vi "NEW数据采集传输系统.vi"() -> ()   [LabVIEW 2016, in "数据传输系统.lvlib"]
uses:
  <vilib>/Averna/Notify Icon/NotifyIcon.llb/BalloonIcon.ctl
  <vilib>/Utility/miscctls.llb/LVPointTypeDef.ctl
  <vilib>/Utility/config.llb/Read Key (String).vi
  <vilib>/Averna/Notify Icon/NotifyIcon.llb/GetSelectedItemEvent.vi
  <vilib>/Averna/Notify Icon/NotifyIcon.llb/SetVisible.vi
  <vilib>/Averna/Notify Icon/NotifyIcon.llb/SetMenuDefaultItem.vi
  <vilib>/Averna/Notify Icon/NotifyIcon.llb/SetTipText.vi
  <vilib>/Utility/config.llb/NI_LVConfig.lvlib
  data/FreeMem.dll
  <vilib>/Averna/Notify Icon/NotifyIcon.llb/NotifyIcon.lvclass
  <vilib>/ptbypt/NI_PtbyPt.lvlib
panel:
  in  "参数数值":T1={"CODMn"=TRUE, "CODCr"=TRUE, "DO"=TRUE, "铜"=TRUE, "PH"=TRUE, "氨氮"=TRUE, "比电导率"=TRUE, "水温"=TRUE, "COD"=TRUE, "浊度"=TRUE, "总氮"=TRUE, "总磷"=TRUE, "叶绿素a"=TRUE, "藻密度"=TRUE, "水位"=TRUE, "流速"=TRUE, "瞬时流量"=TRUE, "累积流量"=TRUE, "亚硝酸盐"=TRUE, "硫化物"=TRUE, "ORP"=TRUE, "铅"=TRUE, "镉"=TRUE, "锌"=TRUE, "镍"=TRUE, "锰"=TRUE, "汞"=TRUE, "气温"=TRUE, "气压"=TRUE, "风速"=TRUE, "风向"=TRUE}
  in  "配置表":bool caption="确定"
  out "配置表格":string[][](table)
  in  "updateconfiguration":T2={"主机"="27.154.58.30", "用户"="update", "密码"="std23506", "远程路径"="数据传输系统\\平台数据传输系统.exe", "下载文件名"="平台数据传输系统.exe", "软件版本"=""}
  out "标题显示":string
  in  "更新":bool
  out "错误输出":errorcluster
  in  "系统编码选择框":string(combo)="地表水质量监测"
  in  "数据发送通道":enum16{"TCP", "VISA"}(ring)
  in  "baud rate":u32=9600 caption="波特率"
  in  "VISA resource name":refnum<visa-resource-name> caption="VISA资源名称"
  in  "实时数据发送时间间隔/min":i32=1
  in  "数据组合发送":bool
  in  "日志、参数发送":bool
  in  "2011发送":bool
  in  "判断数据反馈":bool
  in  "数据发送协议":enum16{"2005-212协议", "2017-212协议"}(ring)=enum."2017-212协议"
  in  "重发时间":T3(ring)
  in  "重发日期":T4(ring)
  in  "开机启动":bool
  in  "确定更改起始时间":bool
  in  "更改起始时间":bool
  in  "数据发送起始时间":timestamp format="%<%.3X\n%Y/%m/%d>T"
  in  "每周自动重发":bool=TRUE
  in  "确定":bool
  in  "返回":bool
  in  "PW":string
  in  "MN":string
  in  "PORT":string
  in  "IP":string
  in  "站点设备":string
  in  "站点名称":string
  out "设置超时时间/min":i32=1
  out "状态信息":T5={"1st Error to Convert "=63, "步骤 "=enum."发送数据", "元素"="实时数据", "TCP服务端掉线计数"=0, "TCP掉线时间节点"="2019/05/08 15:24:17"} {"1st Error to Convert" items=["无错误", "参数错误", "内存已满", "超出区域", "文件结束", "文件已打开", "一般文件IO错误", "未找到文件", "文件权限错误", "磁盘已满", "路径副本", "打开过多文件", "未启用", "未找到资源文件", "无法添加资源", "未找到资源", "未找到图像", "图像内存错误", "画笔不存在", "配置错误类型", "配置未找到解析段", "配置解析错误", "配置内存错误", "错误外部代码格式", "错误外部代码偏移量", "外部代码不存在", "空窗口", "销毁窗口错误", "空菜单", "打印已中止", "错误打印记录", "打印驱动程序错误", "打印时窗口错误", "打印时内存错误", "打印对话框错误", "一般打印错误", "无效设备引用句柄", "设备未找到", "设备参数错误", "设备单位错误", "无法打开设备", "设备调用已中止", "一般错误", "用户已取消", "对象ID过低", "对象ID过高", "对象不在堆中", "未知的堆", "错误DefProc ID", "DefProc不在表格中", "范围外信息", "空方法", "未知信息", "不支持管理器调用", "错误地址", "连接过程中", "连接超时", "连接过程中", "不支持网络属性", "网络错误", "正在使用的地址", "系统缺少内存", "连接已中止", "连接已拒绝", "连接未建立", "连接已建立", "连接已关闭", "初始化错误（交互应用程序管理器）", "错误事件发生", "等待无约束事件发生处理程序", "事件发生队列溢出", "错误路径", "未发出信号量", "未识别类型（交互应用程序管理器）"]}
  out "数据接收超时指示灯":bool
  out "空闲时间/s":string
  out "系统时间":string
  out "实时小时数据上传":bool
  out "系统状态改变":bool
  out "软件版本":string
  out "掉线指示":bool
  out "核查数据上传":bool
  out "配置信息":T6
  in  "参数配置":bool
  out "反控数据发送":bool
  out "读取报文显示":string
  out "发送报文显示":string
  out "心跳包":bool
  out "通信状态":bool
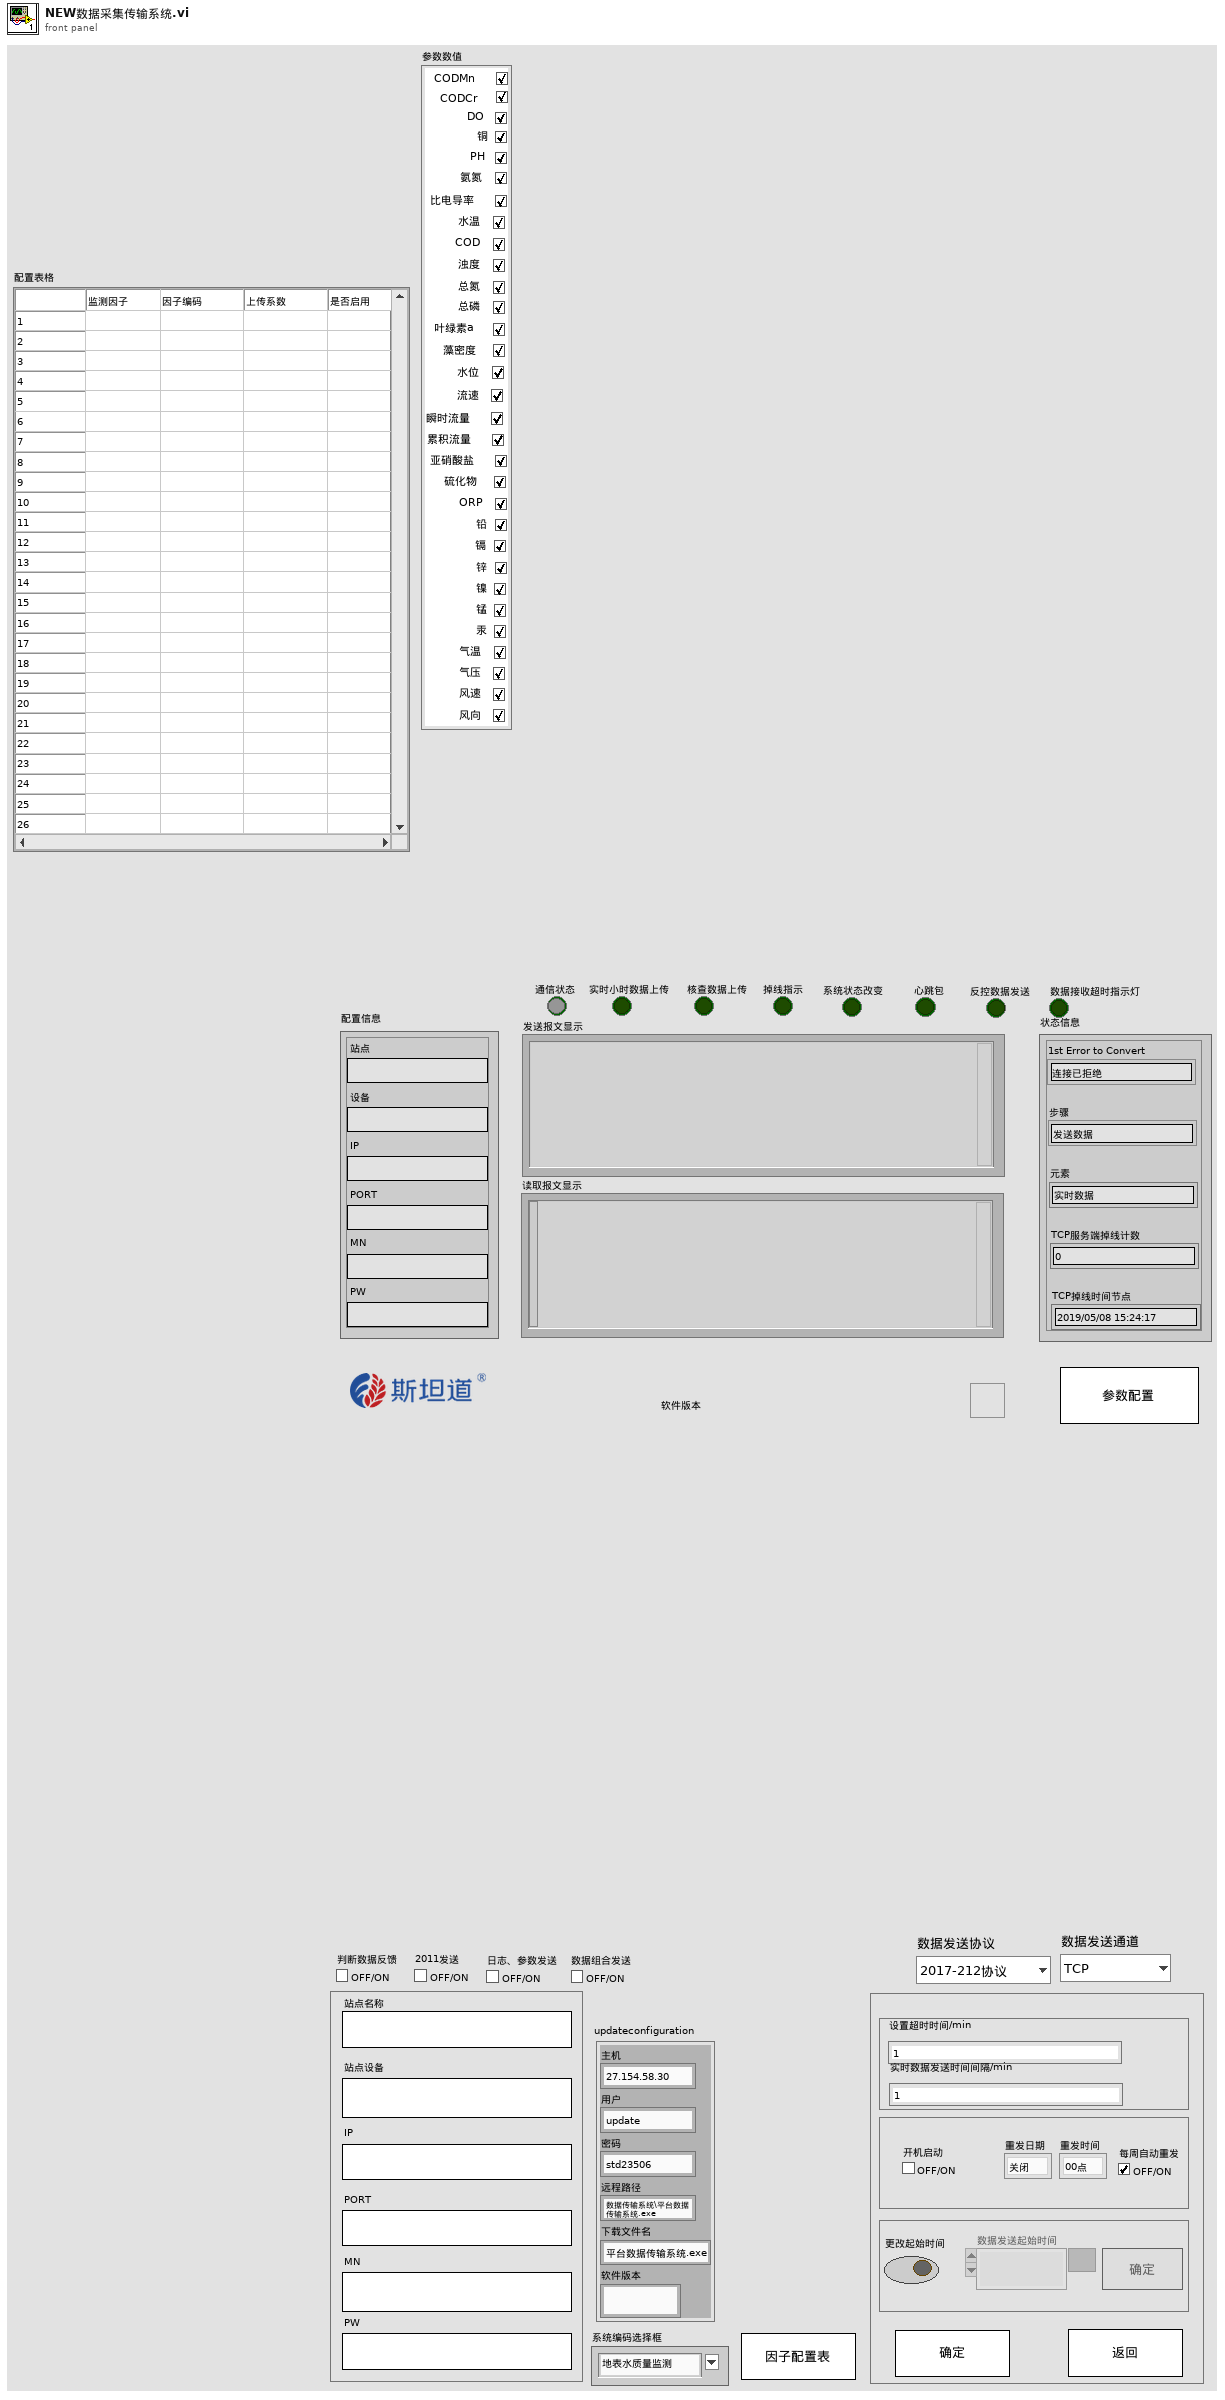
[diagram p1: front panel]
types:
  T1 = cluster{"CODMn":bool, "CODCr":bool, "DO":bool, "铜":bool, "PH":bool, "氨氮":bool, "比电导率":bool, "水温":bool, "COD":bool, "浊度":bool, "总氮":bool, "总磷":bool, "叶绿素a":bool, "藻密度":bool, "水位":bool, "流速":bool, "瞬时流量":bool, "累积流量":bool, "亚硝酸盐":bool, "硫化物":bool, "ORP":bool, "铅":bool, "镉":bool, "锌":bool, "镍":bool, "锰":bool, "汞":bool, "气温":bool, "气压":bool, "风速":bool, "风向":bool}
  T2 = cluster{"主机":string, "用户":string, "密码":string, "远程路径":string, "下载文件名":string, "软件版本":string}
  T3 = enum16{"00点", "01点", "02点", "03点", "04点", "05点", "06点", "07点", "08点", "09点", "10点", "11点", "12点", "13点", "14点", "15点", "16点", "17点", "18点", "19点", "20点", "21点", "22点", "23点"}
  T4 = enum16{"关闭", "星期日", "星期一", "星期二", "星期三", "星期四", "星期五", "星期六"}
  T5 = cluster{"1st Error to Convert ":i32, "步骤 ":enum16{"打开连接", "发送数据", "读取数据", "数据处理", "关闭连接"}, "元素":string, "TCP服务端掉线计数":i32, "TCP掉线时间节点":string}
  T6 = cluster{"站点":string, "设备":string, "IP":string, "PORT":string, "MN":string, "PW":string}
  T7 = enum32{"Invalid", "Standard", "Closed", "Hidden", "Minimized", "Maximized"}
  T8 = typedef "LVDateTimeRec.ctl" = cluster{"秒数的小数部分":dbl, "秒":i32, "分":i32, "时":i32, "日":i32, "月":i32, "年":i32, "天数（周）":i32, "天数（年）":i32, "DST":i32}
  T9 = typedef "LVPointTypeDef.ctl" = cluster{"Horizontal":i16, "Vertical":i16}
  T10 = cluster{"CODMn":string, "CODCr":string, "DO":string, "铜":string, "PH":string, "氨氮":string, "比电导率":string, "水温":string, "COD":string, "浊度":string, "总氮":string, "总磷":string, "叶绿素a":string, "藻密度":string, "水位":string, "流速":string, "瞬时流量":string, "累积流量":string, "亚硝酸盐":string, "硫化物":string, "ORP":string, "铅":string, "镉":string, "锌":string, "镍":string, "锰":string, "汞":string, "气温":string, "气压":string, "风速":string, "风向":string}
  T11 = typedef "NI_LVConfig.lvlib/Config Data RefNum.ctl" = refnum<k1>
  T12 = typedef "imagedata.ctl" = cluster{"image type":i32, "image depth":i32, "image":u8[], "mask":u8[], "colors":u32[], "Rectangle":cluster{"left":i16, "top":i16, "right":i16, "bottom":i16}}
  T13 = cluster{"[0]":string, "[1]":string, "[2]":string, "[3]":string, "[4]":string, "[5]":string, "[6]":string, "[7]":string, "[8]":string, "[9]":string, "[10]":string, "[11]":string, "[12]":string, "[13]":string, "[14]":string, "[15]":string, "[16]":string, "[17]":string, "[18]":string, "[19]":string, "[20]":string, "[21]":string, "[22]":string, "[23]":string, "[24]":string, "[25]":string, "[26]":string, "[27]":string, "[28]":string, "[29]":string, "[30]":string}
  T14 = enum8{"Enabled", "Disabled", "Disabled and Grayed Out"}
  T15 = cluster{"配置表格[0]":string, "配置表格[1]":string, "配置表格[2]":string, "配置表格[3]":string, "配置表格[4]":string, "配置表格[5]":string, "配置表格[6]":string, "配置表格[7]":string, "配置表格[8]":string, "配置表格[9]":string, "配置表格[10]":string, "配置表格[11]":string, "配置表格[12]":string, "配置表格[13]":string, "配置表格[14]":string, "配置表格[15]":string, "配置表格[16]":string, "配置表格[17]":string, "配置表格[18]":string, "配置表格[19]":string, "配置表格[20]":string, "配置表格[21]":string, "配置表格[22]":string, "配置表格[23]":string, "配置表格[24]":string, "配置表格[25]":string, "配置表格[26]":string, "配置表格[27]":string, "配置表格[28]":string, "配置表格[29]":string, "配置表格[30]":string}
  T16 = cluster{"[0]":string, "[1]":string, "[2]":string, "[3]":string, "[4]":string, "[5]":string, "[6]":string, "[7]":string}
  T17 = cluster{"[0]":string, "[1]":string, "[2]":string, "[3]":string, "[4]":string, "[5]":string, "[6]":string, "[7]":string, "[8]":string, "[9]":string, "[10]":string, "[11]":string, "[12]":string, "[13]":string, "[14]":string}
  T18 = typedef "NotifyIcon.lvlib/NotifyIcon.lvclass/BalloonIcon.ctl" = enum32{"None", "Information", "Warning", "Error"}
  T19 = enum32{"invalid app kind", "Development System", "Run Time System", "Student Edition", "Embedded LabVIEW", "Evaluation", "Custom"}
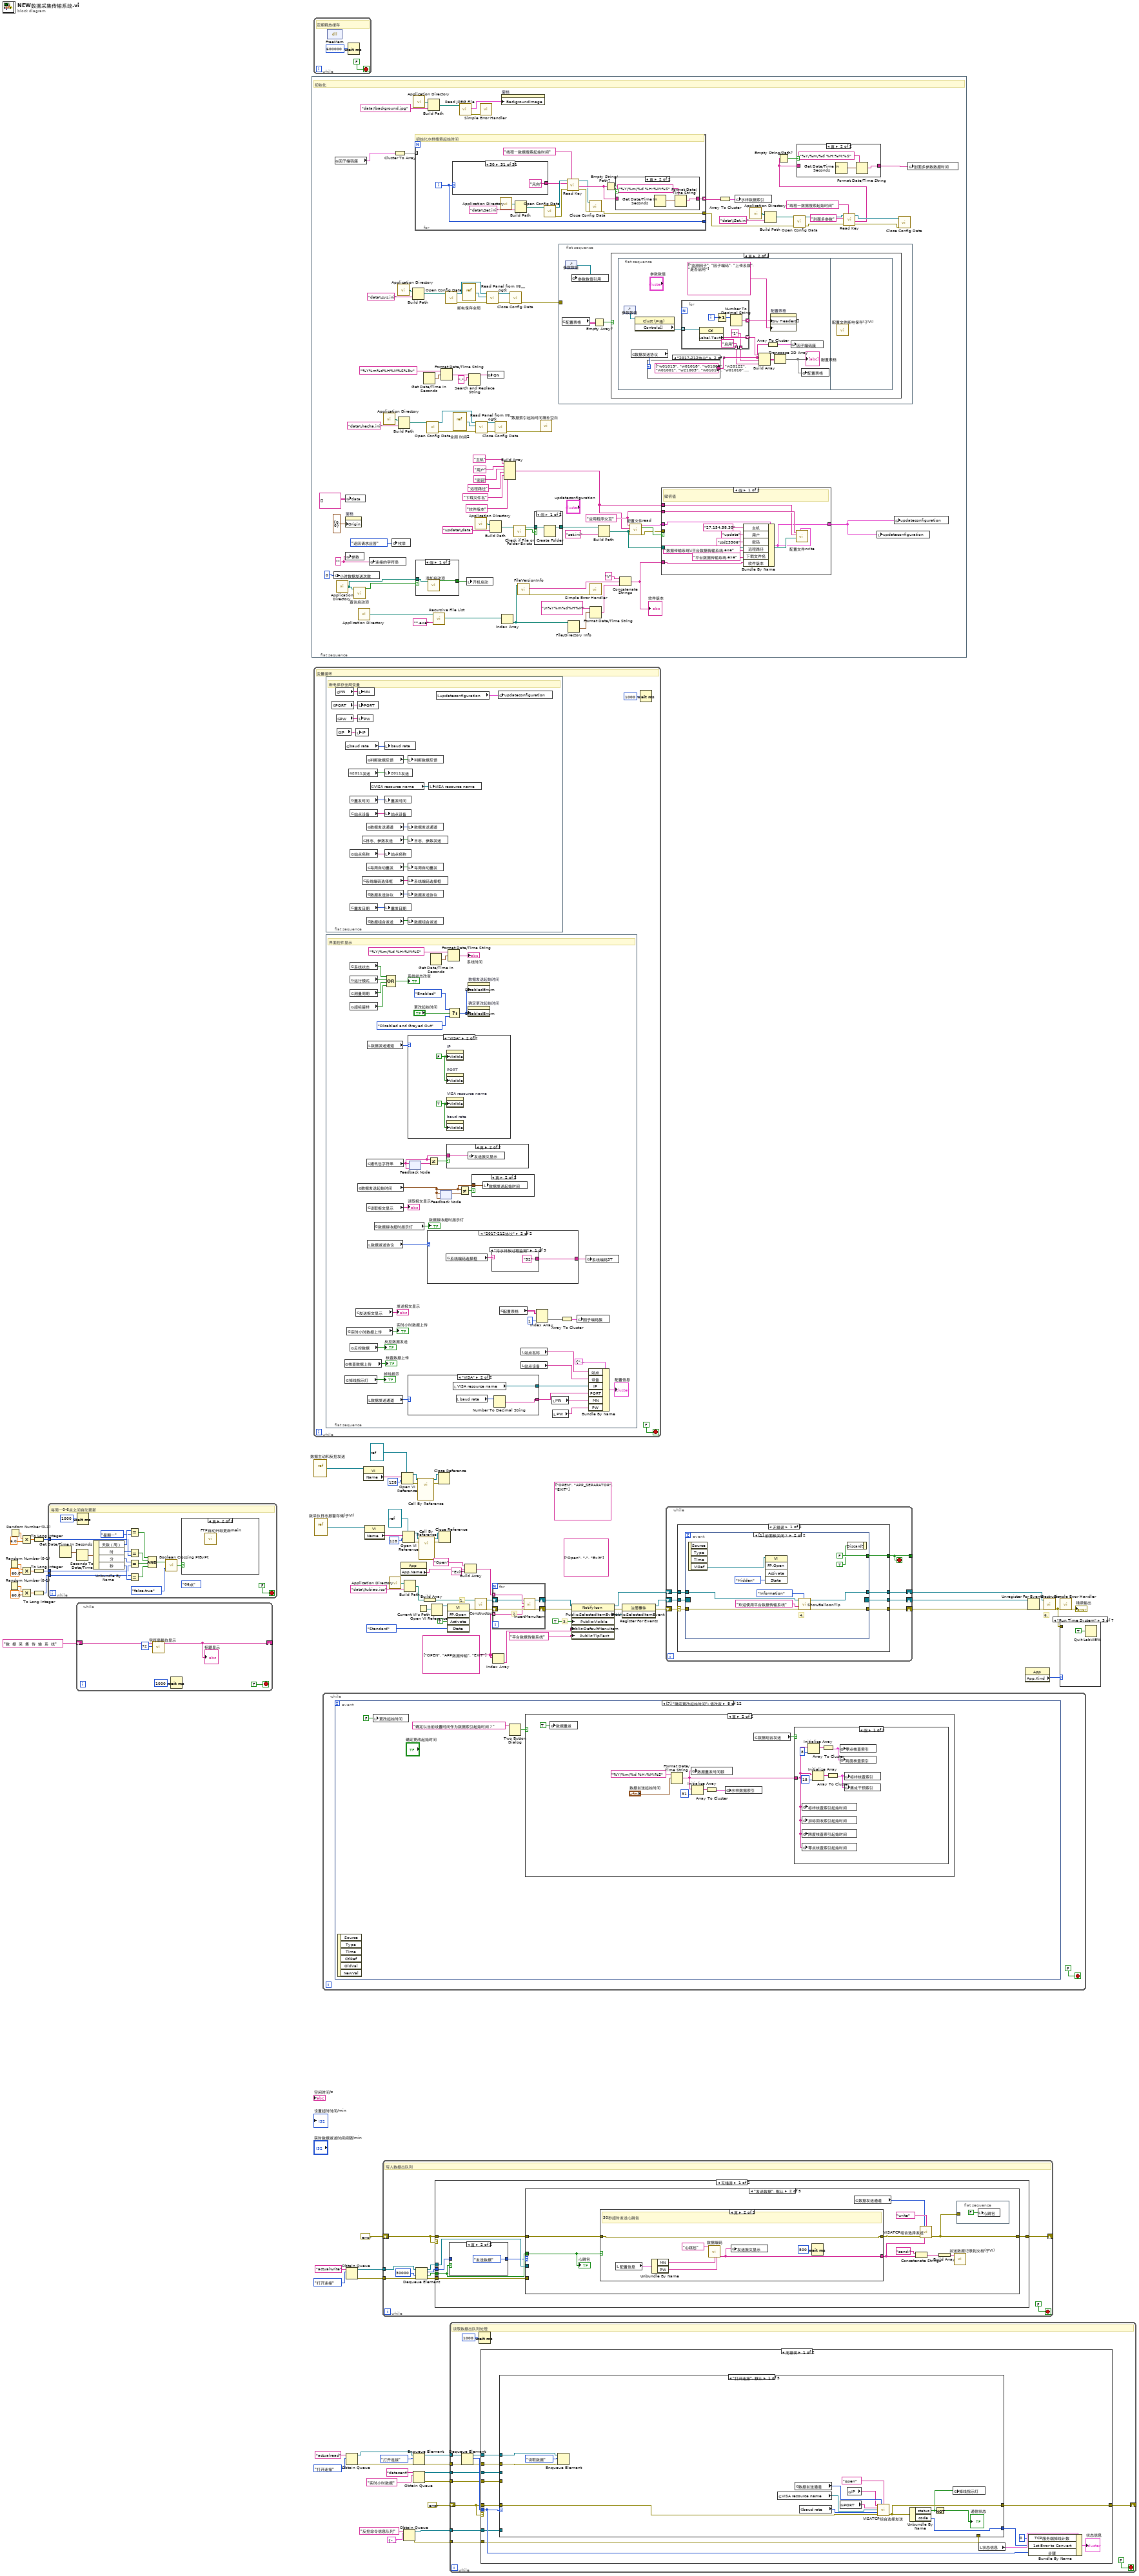
[diagram p0: block diagram]
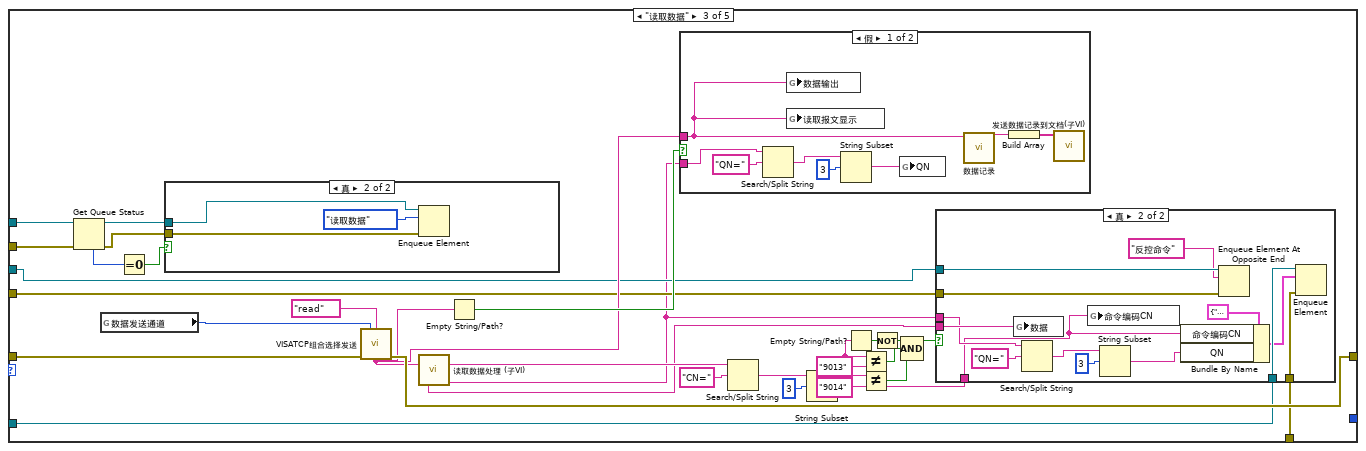
[diagram p4: hidden frame]
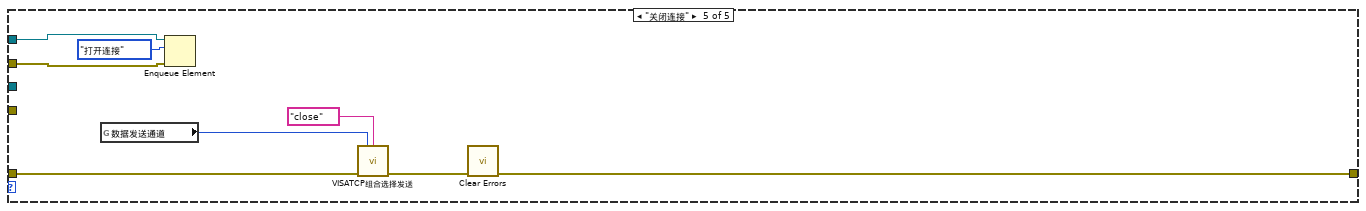
[diagram p9: hidden frame]
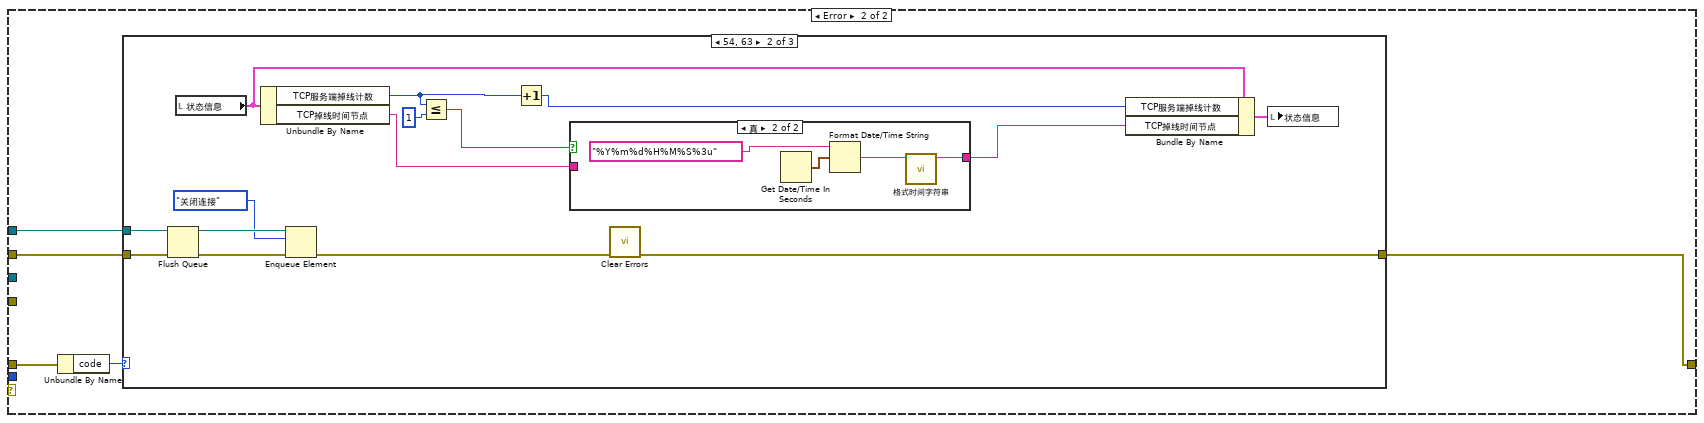
[diagram p10: hidden frame]
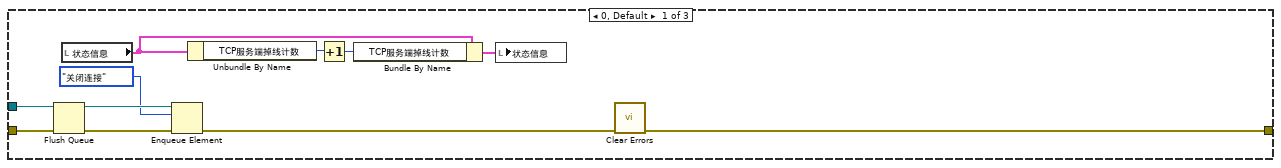
[diagram p11: hidden frame]
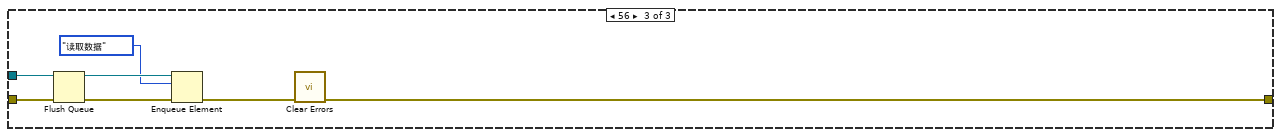
[diagram p13: hidden frame]
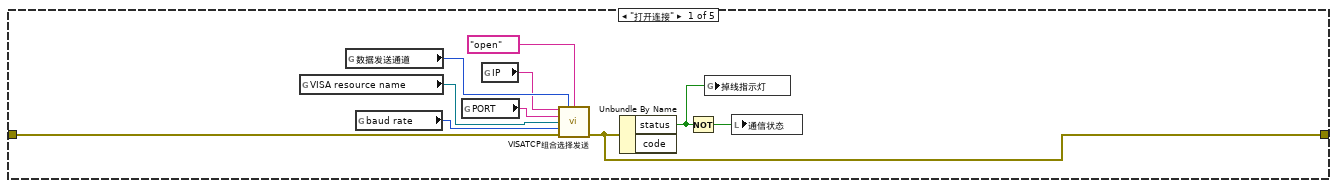
[diagram p15: hidden frame]
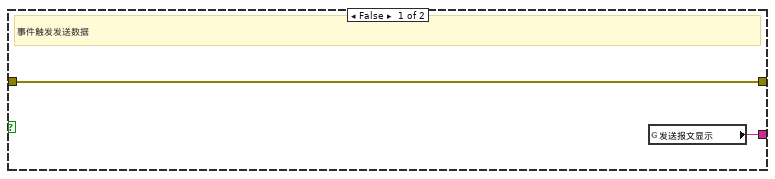
[diagram p16: hidden frame]
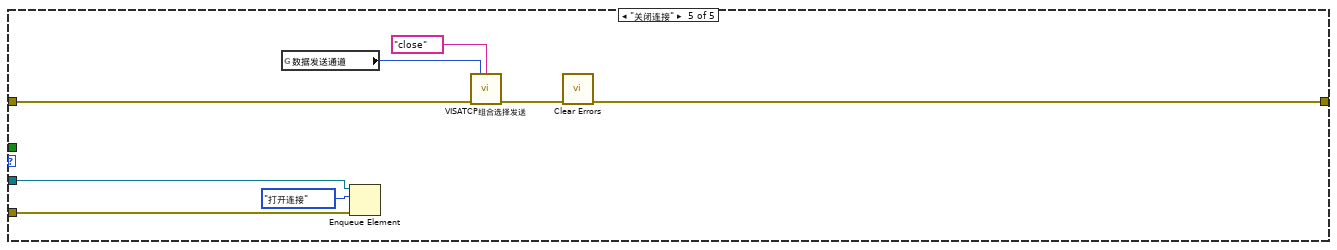
[diagram p19: hidden frame]
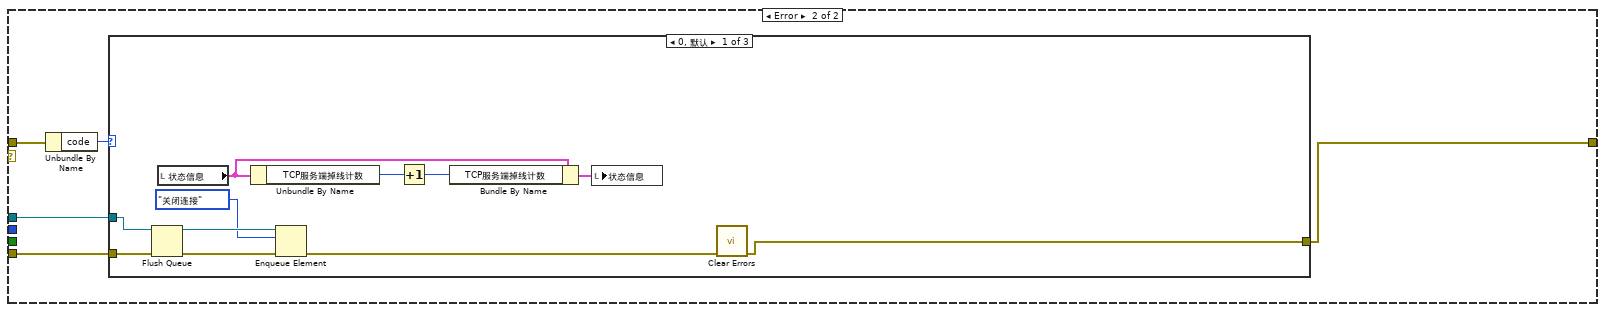
[diagram p20: hidden frame]
diagram:
  w1 = string[] ["OPEN", "APP数据传输", "EXIT"]
  (unwired) string[] ["OPEN", "APP_SEPARATOR", "EXIT"]
  (unwired) string[] ["Open", "-", "Exit"]
  # "6."
  # "3."
  # "1."
  n1 = Random Number (0-1)() -> (number: 0 to 1=w15:dbl)
  n2 = Random Number (0-1)() -> (number: 0 to 1=w14:dbl)
  n3 = Random Number (0-1)() -> (number: 0 to 1=w18:dbl)
  n4 = Multiply(x=w18, y=6.0) -> (x*y=w12:dbl)
  n5 = Multiply(x=w15, y=60.0) -> (x*y=w10:dbl)
  n6 = Multiply(x=w14, y=60.0) -> (x*y=w8:dbl)
  n7 = To Long Integer(number=w12) -> (32bit integer=w11:i32)
  n8 = To Long Integer(number=w10) -> (32bit integer=w9:i32)
  n9 = To Long Integer(number=w8) -> (32bit integer=w7:i32)
  n10 = while {
    tunnel: w11 -> [w91]
    tunnel: w9 -> [w86]
    tunnel: w7 -> [w85]
    stop <- FALSE stop-if-true
    (unwired) T3."06点" ("重发时间")
    # "每周一0-6点之间自动更新"
    n11 = Get Date/Time In Seconds() -> (seconds since 1Jan1904=w100:timestamp)
    n12 = Seconds To Date/Time(time stamp (now)=w100) -> (date time rec=w96:T8)  [unwired: 1 in]
    n13 = Wait (ms)(milliseconds to wait=u32 1000 ("等待时间（毫秒）")) -> ()  [unwired: 1 out]
    n14 = Unbundle By Name(w96) -> ("天数（周）"=w99:i32, "时"=w93:i32, "分"=w90:i32, "秒"=w88:i32)
    n15 = Equal?(x=w99, y=T4."星期一" ("重发日期")) -> (x = y?=w98:bool)
    n16 = Equal?(x=w93, y=w91) -> (x = y?=w97:bool)
    n17 = Equal?(x=w90, y=w86) -> (x = y?=w89:bool)
    n18 = Equal?(x=w85, y=w88) -> (x = y?=w87:bool)
    n19 = Compound Arithmetic op=AND ("复合运算")(w98, w97, w89, w87) -> (w95:bool)
    n20 = call <vilib>:"Boolean Crossing PtByPt.vi"("direction"=enum16{"either", "false-true", "true-false"}."false-true", "input"=w95) -> ("crossing"=w84:bool)  [unwired: 1 in]
    n21 = case shown="真" w84 {
      frame False {
      }
      frame True {
        n22 = call "FTP自动升级更新main.vi"() -> ()  [unwired: 12 in]
      }
    }
  }
  n23 = while {
    shift-right: [w104] -> _
    shift-left: "数  据  采  集  传  输  系  统" ("标题显示") -> [w105]
    stop <- FALSE stop-if-true
    n24 = call "字符串移位显示.vi"("字符框大小"=72, "字符串输入"=w105) -> ("移位后字符串"=w104:string)  [unwired: 8 in, 1 out]
    "标题显示" <- w104
    n25 = Wait (ms)(milliseconds to wait=u32 1000 ("等待时间（毫秒）")) -> ()  [unwired: 1 out]
  }
  n26 = flat-sequence {
    frame #0 {
      w142 = "应用程序交互" ("section")
      w189 = "" ("参数")
      # "初始化"
      n27 = global write "全局 小时数据发送次数.vi" "小时数据发送次数"(0 ("数值")) -> ()
      n28 = global read "断电保存全局.vi" "因子编码簇"() -> (w108:T10)
      n29 = call <vilib>:"Application Directory.vi"() -> ("Application Directory"=w111:path)
      n30 = global write "全局 实时数据参数.vi" "data"(string[][] [] ("data")) -> ()
      n31 = property on="窗格" class="Pane"("Origin"=T9 {"Horizontal"=0, "Vertical"=0} ("原点")) -> ()  [unwired: 2 in, 2 out]
      n32 = global write "全局 实时数据参数.vi" "参数"(w189) -> ()
      n33 = call "查询启动项.vi"("启动文件路径"=w111) -> ("包含启动项"=w112:bool)  [unwired: 9 in, 1 out]
      n34 = call <vilib>:"Application Directory.vi"() -> ("Application Directory"=w169:path)
      n35 = global write "全局 实时数据参数.vi" "连接的字符串"(w189) -> ()
      n36 = call <vilib>:"Application Directory.vi"() -> ("Application Directory"=w155:path)
      n37 = global write "全局1.vi" "枚举"(enum16{"返回请求应答", "上传数据", "返回执行结果"}."返回请求应答" ("枚举")) -> ()
      n38 = Cluster To Array(cluster=w108) -> (array=w148:string[])
      n39 = call <vilib>:"Application Directory.vi"() -> ("Application Directory"=w163:path)
      n40 = Build Path(base path=w155, name or relative path="data\\hecha.ini" ("名称或相对路径")) -> (appended path=w157:path)
      n41 = Build Path(base path=w163, name or relative path="data\\sys.ini" ("名称或相对路径")) -> (appended path=w161:path)
      n42 = call <vilib>:"Application Directory.vi"() -> ("Application Directory"=w180:path)
      n43 = for {
        tunnel: w148 -> [_] mode=indexing
        tunnel: [w248] -> _
        tunnel: [w245] -> w147 mode=indexing
        tunnel: [w244] -> w122
        i -> [w248]
        # "初始化水样搜索起始时间"
        n44 = case shown="30" w248 {
          tunnel: ["CODMn" "CODCr" "DO" "铜" "PH" "氨氮" "比电导率" "水温" "COD" "浊度" "总氮" "总磷" "叶绿素a" "藻密度" "水位" "流速" "瞬时流量" "累积流量" "亚硝氮" "硫化物" "ORP" "铅" "镉" "锌" "镍" "锰" "汞" "气温" "气压" "风速" "风向"] -> w251
          frame 0, Default {
          }
          frame 1 {
          }
          frame 2 {
          }
          frame 3 {
          }
          frame 4 {
          }
          frame 5 {
          }
          frame 6 {
          }
          frame 7 {
          }
          frame 8 {
          }
          frame 9 {
          }
          frame 10 {
          }
          frame 11 {
          }
          frame 12 {
          }
          frame 13 {
          }
          frame 14 {
          }
          frame 15 {
          }
          frame 16 {
          }
          frame 17 {
          }
          frame 18 {
          }
          frame 19 {
          }
          frame 20 {
          }
          frame 21 {
          }
          frame 22 {
          }
          frame 23 {
          }
          frame 24 {
          }
          frame 25 {
          }
          frame 26 {
          }
          frame 27 {
          }
          frame 28 {
          }
          frame 29 {
          }
          frame 30 {
          }
        }
        n45 = call <vilib>:"Application Directory.vi"() -> ("Application Directory"=w257:path)
        n46 = Build Path(base path=w257, name or relative path="data\\Set.ini" ("名称或相对路径")) -> (appended path=w255:path)
        n47 = call <vilib>:"Open Config Data.vi"("configuration file path"=w255) -> ("error out"=w253:errorcluster, "refnum"=w254:T11)  [unwired: 8 in, 1 out]
        n48 = call-poly <vilib>:"Read Key.vi"("section"="线程一数据搜索起始时间", "error in (no error)"=w253, "key"=w251, "refnum"=w254) -> ("error out"=w246:errorcluster, "value"=w249:string, "refnum out"=w247:T11)  [unwired: 4 in, 1 out]
        n49 = call <vilib>:"Close Config Data.vi"("error in (no error)"=w246, "refnum"=w247) -> ("error out"=w244:errorcluster)  [unwired: 8 in, 1 out]
        n50 = Empty String/Path?(string/path=w249) -> (empty?=w250:bool)
        n51 = case shown="真" w250 {
          tunnel: [w258 w259] -> w245
          tunnel: w249 -> [w258 _]
          frame False {
          }
          frame True {
            n52 = Get Date/Time In Seconds() -> (seconds since 1Jan1904=w261:timestamp)
            n53 = Format Date/Time String(time format string (%c)="%Y/%m/%d %H:%M:%S" ("时间格式字符串(%c)"), seconds (now)=w261) -> (date/time string=w259:string)  [unwired: 1 in]
          }
        }
      }
      n54 = case shown="假" w112 {
        selector: w112 -> [_ w218]
        tunnel: w111 -> [w217 _]
        tunnel: [w216 w218] -> w110
        frame False {
          n55 = call "添加启动项.vi"("启动文件路径"=w217) -> ("添加成功标记"=w216:bool)  [unwired: 9 in, 1 out]
        }
        frame True {
        }
      }
      n56 = Get Date/Time In Seconds() -> (seconds since 1Jan1904=w185:timestamp)
      n57 = call <vilib>:"Open Config Data.vi"("configuration file path"=w157) -> ("error out"=w151:errorcluster, "refnum"=w152:T11)  [unwired: 8 in, 1 out]
      n58 = Build Path(base path=w180, name or relative path="data\\background.jpg" ("名称或相对路径")) -> (appended path=w179:path)
      n59 = call <vilib>:"Recursive File List.vi"("pattern"="*.exe", "Folder Path"=w169) -> ("All Files in Dir"=w175:path[])  [unwired: 5 in, 4 out]
      n60 = Format Date/Time String(time format string (%c)="%Y%m%d%H%M%S%3u" ("时间格式字符串(%c)"), seconds (now)=w185) -> (date/time string=w184:string)  [unwired: 1 in]
      n61 = call <vilib>:"Open Config Data.vi"("configuration file path"=w161) -> ("error out"=w167:errorcluster, "refnum"=w166:T11)  [unwired: 8 in, 1 out]
      n62 = vi-ref "全局 时间2.vi"() -> (w153:refnum<vi>)
      n63 = call <vilib>:"Read JPEG File.vi"("path to JPEG file"=w179) -> ("error out"=w177:errorcluster, "image data"=w178:T12)  [unwired: 8 in, 1 out]
      n64 = vi-ref "断电保存全局.vi"() -> (w165:refnum<vi>)
      n65 = local write "开机启动"(w110) -> ()
      n66 = Search and Replace String(input string=w184, search string="." ("搜索字符串")) -> (result string=w182:string)  [unwired: 6 in, 3 out]
      n67 = call <vilib>:"Application Directory.vi"() -> ("Application Directory"=w128:path)
      n68 = call <userlib>:"Read Panel from INI__ogtk.vi"("error in (no error)"=w151, "VI ref"=w153, "refnum"=w152) -> ("error out"=w150:errorcluster, "refnum out"=w154:T11)  [unwired: 7 in]
      n69 = call <vilib>:"Simple Error Handler.vi"("error in (no error)"=w177) -> ()  [unwired: 4 in, 5 out]
      n70 = call <userlib>:"Read Panel from INI__ogtk.vi"("error in (no error)"=w167, "VI ref"=w165, "refnum"=w166) -> ("error out"=w160:errorcluster, "refnum out"=w164:T11)  [unwired: 7 in]
      n71 = global write "全局1.vi" "QN"(w182) -> ()
      n72 = Build Path(base path=w128, name or relative path="update\\data" ("名称或相对路径")) -> (appended path=w129:path)
      n73 = call <vilib>:"Close Config Data.vi"("error in (no error)"=w150, "refnum"=w154) -> ("error out"=w149:errorcluster)  [unwired: 8 in, 1 out]
      n74 = property on="窗格" class="Pane"("BackgroundImage"=w178) -> ()  [unwired: 2 in, 2 out]
      n75 = Index Array(array=w175) -> (element=w174:path)  [unwired: 1 in]
      n76 = Build Array("主机" ("section"), "用户" ("section"), "密码" ("key"), "远程路径" ("key"), "下载文件名" ("key"), "软件版本" ("key")) -> (w132:string[])
      n77 = call <vilib>:"Close Config Data.vi"("error in (no error)"=w160, "refnum"=w164) -> ("error out"=w109:errorcluster)  [unwired: 8 in, 1 out]
      n78 = call <vilib>:"Check if File or Folder Exists.vi"("path"=w129) -> ("file or folder exists?"=w130:bool, "dup path"=w131:path)  [unwired: 8 in, 1 out]
      n79 = call <vilib>:"FileVersionInfo.vi"("Application Path in"=w174) -> ("error out"=w168:errorcluster, "File Version Info"=w158:string)  [unwired: 7 in, 2 out]
      n80 = case shown="假" w130 {
        tunnel: w131 -> [w224 w225]
        tunnel: [w223 w225] -> w126
        frame False {
          n81 = Create Folder(path (use dialog)=w224) -> (created path=w223:path)  [unwired: 2 in, 2 out]
        }
        frame True {
        }
      }
      n82 = call "数据索引起始时间填补空白.vi"("error in (no error)"=w149) -> ()  [unwired: 10 in, 1 out]
      n83 = flat-sequence {
        tunnel: w109 -> [_]
        frame #0 {
          n84 = global read "断电保存全局.vi" "配置表格"() -> (w194:string[][])
          n85 = control-ref of="参数数值"() -> (w192:refnum<vi>)
          n86 = global write "断电保存全局.vi" "参数数值引用"(w192) -> ()
          n87 = Empty Array?(array=w194) -> (empty?=w193:bool)
          n88 = case shown="真" w193 {
            frame False {
            }
            frame True {
              n89 = flat-sequence {
                frame #0 {
                  n90 = control-ref of="参数数值"() -> (w195:refnum<vi>)
                  n91 = global read "断电保存全局.vi" "数据发送协议"() -> (w200:enum16{"2005-212协议", "2017-212协议"})
                  n92 = property on="属性节点" class="Clust (严格)"(reference=w195) -> ("Controls[]"=w202:refnum<vi>[])  [unwired: 1 in, 2 out]
                  n93 = case shown="\"2017-212协议\"" w200 {
                    tunnel: [string[] ["w01019", "011", "w01009", "w20122", "001", "060", "w01014", "w01010", "w01018", "w01003", "065", "101", "w01016", "w19011", "e01201", "e01202", "B01", "e01204", "w21006", "w21019", "w01100", "w20120", "w20115", "w20123", "w20121", "w20124", "w20111"] string[] ["w01019", "w01018", "w01009", "w20122", "w01001", "w21003", "w01014", "w01010", "w01018", "w01003", "w21001", "w21011", "w01016", "w19011", "e01201", "e01202", "e01203", "e01204", "w21006", "w21019", "w01100", "w20120", "w20115", "w20123", "w20121", "w20124", "w20111"]] -> w198
                    frame "2005-212协议", Default {
                    }
                    frame "2017-212协议" {
                    }
                  }
                  n94 = for {
                    tunnel: w202 -> [w215] mode=indexing
                    tunnel: [w214] -> w204 mode=indexing
                    tunnel: [w212] -> w203 mode=indexing
                    tunnel: ["1"] -> w197 mode=indexing
                    tunnel: ["启用"] -> w196 mode=indexing
                    i -> [w213]
                    n95 = property class="Ctl"(reference=w215) -> ("Label.Text"=w214:string)  [unwired: 1 in, 2 out]
                    n96 = Increment(x=w213) -> (x+1=w211:i32)
                    n97 = Number To Decimal String(number=w211) -> (decimal integer string=w212:string)  [unwired: 1 in]
                  }
                  n98 = Build Array(w204, w198, w197, w196) -> (w206:string[][])
                  n99 = Array To Cluster(array=w198) -> (cluster=w199:T13)
                  n100 = property on="配置表格" class="Tbl (严格)"("Row Headers[]"=w203, "Column Headers[]"=string[] ["监测因子", "因子编码", "上传系数", "是否启用"]) -> ()  [unwired: 2 in, 2 out]
                  n101 = Transpose 2D Array(2D array=w206) -> (transposed array=w201:string[][])
                  "配置表格" <- w201
                  n102 = global write "断电保存全局.vi" "因子编码簇"(w199) -> ()
                  n103 = global write "断电保存全局.vi" "配置表格"(w201) -> ()
                }
                frame #1 {
                  n104 = call "配置文件断电保存(子VI).vi"() -> ()  [unwired: 12 in]
                }
              }
            }
          }
        }
      }
      n105 = File/Directory Info(path=w174) -> (last mod=w173:timestamp)  [unwired: 1 in, 6 out]
      n106 = call <vilib>:"Simple Error Handler.vi"("error in (no error)"=w168) -> ()  [unwired: 4 in, 5 out]
      n107 = Format Date/Time String(time format string (%c)="\n%Y%m%d%H%M" ("时间格式字符串(%c)"), seconds (now)=w173) -> (date/time string=w170:string)  [unwired: 1 in]
      n108 = Build Path(base path=w126, name or relative path="set.ini" ("名称或相对路径")) -> (appended path=w141:path)
      n109 = Concatenate Strings("V" ("字符串"), w158, w170) -> (w143:string)
      "软件版本" <- w143
      n110 = call "配置文件read.vi"("configuration file path"=w141, "键数组"=w132, "段"=w142) -> ("error out"=w140:errorcluster, "section exists?"=w145:bool, "updateconfiguration"=w144:T2)  [unwired: 6 in]
      n111 = case shown="假" w145 {
        tunnel: w144 -> [w232 w238]
        tunnel: [w231 w237] -> w139
        tunnel: w143 -> [w226 w243]
        tunnel: w142 -> [w235 w242]
        tunnel: w132 -> [w234 w241]
        tunnel: w141 -> [w233 w240]
        tunnel: w140 -> [_ w239]
        frame False {
          # "赋初值"
          n112 = Bundle By Name(cluster=w232, "主机"="27.154.58.30" ("key"), "用户"="update", "密码"="std23506", "远程路径"="数据传输系统\\平台数据传输系统.exe", "下载文件名"="平台数据传输系统.exe", "软件版本"=w226) -> (w231:T2)
          n113 = call "配置文件write.vi"("updateconfiguration"=w231, "configuration file path"=w233, "键数组"=w234, "段"=w235) -> ()  [unwired: 7 in, 1 out]
        }
        frame True {
          # "本地"
          n114 = Bundle By Name(cluster=w238, "软件版本"=w243) -> (w237:T2)
          n115 = call "配置文件write.vi"("updateconfiguration"=w237, "error in (no error)"=w239, "configuration file path"=w240, "键数组"=w241, "段"=w242) -> ()  [unwired: 6 in, 1 out]
        }
      }
      n116 = Array To Cluster(array=w147) -> (cluster=w146:T13)
      n117 = global write "全局 水样时间.vi" "水样数据索引"(w146) -> ()
      n118 = call <vilib>:"Application Directory.vi"() -> ("Application Directory"=w125:path)
      n119 = Build Path(base path=w125, name or relative path="data\\Set.ini" ("名称或相对路径")) -> (appended path=w123:path)
      n120 = call <vilib>:"Open Config Data.vi"("error in (no error)"=w122, "configuration file path"=w123) -> ("error out"=w119:errorcluster, "refnum"=w120:T11)  [unwired: 7 in, 1 out]
      n121 = call-poly <vilib>:"Read Key.vi"("section"="线程一数据搜索起始时间", "error in (no error)"=w119, "key"="剖面多参数", "refnum"=w120) -> ("error out"=w116:errorcluster, "value"=w114:string, "refnum out"=w117:T11)  [unwired: 4 in, 1 out]
      n122 = Empty String/Path?(string/path=w114) -> (empty?=w113:bool)
      n123 = case shown="真" w113 {
        tunnel: [w219 w220] -> w115
        tunnel: w114 -> [w219 _]
        frame False {
        }
        frame True {
          n124 = Get Date/Time In Seconds() -> (seconds since 1Jan1904=w222:timestamp)
          n125 = Format Date/Time String(time format string (%c)="%Y/%m/%d %H:%M:%S" ("时间格式字符串(%c)"), seconds (now)=w222) -> (date/time string=w220:string)  [unwired: 1 in]
        }
      }
      n126 = local write "updateconfiguration"(w139) -> ()
      n127 = global write "update全局.vi" "updateconfiguration"(w139) -> ()
      n128 = call <vilib>:"Close Config Data.vi"("error in (no error)"=w116, "refnum"=w117) -> ()  [unwired: 8 in, 2 out]
      n129 = global write "全局 水样时间.vi" "剖面多参数数据时间"(w115) -> ()
    }
  }
  n130 = while {
    stop <- FALSE stop-if-true
    # "定期释放缓存"
    n131 = dll-call lib="PTH2aabs F\tgitkrakenCC6平台数采程序 - V2.0.1（正式修改迭代版）dataFreeMem.dll" fn="FreeMem"() -> ()  [unwired: 4 in, 2 out]
    n132 = Wait (ms)(milliseconds to wait=u32 600000 ("等待时间（毫秒）")) -> ()  [unwired: 1 out]
  }
  n133 = while {
    stop <- FALSE stop-if-true
    # "变量循环"
    n134 = flat-sequence {
      frame #0 {
        # "断电保存全局变量"
        n135 = global read "断电保存全局.vi" "PORT"() -> (w370:string)
        n136 = global read "断电保存全局.vi" "MN"() -> (w369:string)
        n137 = global read "断电保存全局.vi" "PW"() -> (w368:string)
        n138 = global read "断电保存全局.vi" "IP"() -> (w371:string)
        n139 = global read "断电保存全局.vi" "baud rate"() -> (w366:u32)
        n140 = global read "断电保存全局.vi" "2011发送"() -> (w362:bool)
        n141 = global read "断电保存全局.vi" "重发时间"() -> (w356:T3)
        n142 = global read "断电保存全局.vi" "站点设备"() -> (w372:string)
        n143 = global read "断电保存全局.vi" "站点名称"() -> (w373:string)
        n144 = global read "断电保存全局.vi" "重发日期"() -> (w364:T4)
        n145 = local write "IP"(w371) -> ()
        n146 = local write "MN"(w369) -> ()
        n147 = local write "PORT"(w370) -> ()
        n148 = local write "PW"(w368) -> ()
        n149 = global read "断电保存全局.vi" "日志、参数发送"() -> (w361:bool)
        n150 = global read "断电保存全局.vi" "系统编码选择框"() -> (w357:string)
        n151 = global read "断电保存全局.vi" "判断数据反馈"() -> (w363:bool)
        n152 = global read "断电保存全局.vi" "数据发送通道"() -> (w358:enum16{"TCP", "VISA"})
        n153 = global read "断电保存全局.vi" "每周自动重发"() -> (w365:bool)
        n154 = global read "断电保存全局.vi" "数据发送协议"() -> (w359:enum16{"2005-212协议", "2017-212协议"})
        n155 = global read "断电保存全局.vi" "数据组合发送"() -> (w360:bool)
        n156 = global read "断电保存全局.vi" "VISA resource name"() -> (w367:refnum<visa-resource-name>)
        n157 = local write "baud rate"(w366) -> ()
        n158 = local write "2011发送"(w362) -> ()
        n159 = local write "重发时间"(w356) -> ()
        n160 = local write "站点设备"(w372) -> ()
        n161 = local write "站点名称"(w373) -> ()
        n162 = local write "重发日期"(w364) -> ()
        n163 = local write "判断数据反馈"(w363) -> ()
        n164 = local write "数据发送通道"(w358) -> ()
        n165 = local write "日志、参数发送"(w361) -> ()
        n166 = local write "每周自动重发"(w365) -> ()
        n167 = local write "系统编码选择框"(w357) -> ()
        n168 = local write "数据发送协议"(w359) -> ()
        n169 = local write "数据组合发送"(w360) -> ()
        n170 = local write "VISA resource name"(w367) -> ()
        n171 = local read "updateconfiguration"() -> (w355:T2)
        n172 = global write "update全局.vi" "updateconfiguration"(w355) -> ()
      }
    }
    n173 = flat-sequence {
      frame #0 {
        # "界面控件显示"
        n174 = global read "全局1.vi" "核查数据上传"() -> (→"核查数据上传":bool)
        n175 = global read "全局 数据发送重叠.vi" "掉线指示灯"() -> (→"掉线指示":bool)
        n176 = global read "全局1.vi" "实时小时数据上传"() -> (→"实时小时数据上传":bool)
        n177 = global read "全局1.vi" "系统状态"() -> (w304:bool)
        n178 = global read "全局1.vi" "运行模式"() -> (w305:bool)
        n179 = global read "全局1.vi" "测量周期"() -> (w306:bool)
        n180 = global read "全局1.vi" "超标留样"() -> (w307:bool)
        n181 = global read "全局1.vi" "反控数据"() -> (→"反控数据发送":bool)
        n182 = global read "全局1.vi" "发送报文显示"() -> (→"发送报文显示":string)
        n183 = global read "全局1.vi" "数据发送起始时间"() -> (w301:timestamp)
        n184 = global read "全局1.vi" "通讯包字符串"() -> (w318:string)
        n185 = global read "全局1.vi" "读取报文显示"() -> (→"读取报文显示":string)
        n186 = local read "数据发送通道"() -> (w312:enum16{"TCP", "VISA"})
        n187 = local read "数据发送协议"() -> (w326:enum16{"2005-212协议", "2017-212协议"})
        n188 = local read "数据发送通道"() -> (w337:enum16{"TCP", "VISA"})
        n189 = global read "全局 数据发送重叠.vi" "数据接收超时指示灯"() -> (→"数据接收超时指示灯":bool)
        n190 = Compound Arithmetic op=OR ("复合运算")(w304, w305, w306, w307) -> (→"系统状态改变":bool)
        n191 = case shown="\"VISA\"" w312 {
          frame "TCP", Default {
            w339 = TRUE ("可见")
            w340 = FALSE ("可见")
            n192 = property on="IP" class="Str"("Visible"=w339) -> ()  [unwired: 2 in, 2 out]
            n193 = property on="PORT" class="Str"("Visible"=w339) -> ()  [unwired: 2 in, 2 out]
            n194 = property on="VISA resource name" class="VISAName"("Visible"=w340) -> ()  [unwired: 2 in, 2 out]
            n195 = property on="baud rate" class="DigNum (严格)"("Visible"=w340) -> ()  [unwired: 2 in, 2 out]
          }
          frame "VISA" {
            w341 = FALSE ("可见")
            w342 = TRUE ("可见")
            n196 = property on="IP" class="Str"("Visible"=w341) -> ()  [unwired: 2 in, 2 out]
            n197 = property on="PORT" class="Str"("Visible"=w341) -> ()  [unwired: 2 in, 2 out]
            n198 = property on="VISA resource name" class="VISAName"("Visible"=w342) -> ()  [unwired: 2 in, 2 out]
            n199 = property on="baud rate" class="DigNum (严格)"("Visible"=w342) -> ()  [unwired: 2 in, 2 out]
          }
        }
        n200 = case shown="\"VISA\"" w337 {
          tunnel: [w351 w354] -> w334
          tunnel: [w350 w352] -> w331
          frame "TCP", Default {
            n201 = local read "PORT"() -> (w350:string)
            n202 = local read "IP"() -> (w351:string)
          }
          frame "VISA" {
            n203 = local read "VISA resource name"() -> (w354:refnum<visa-resource-name>)
            n204 = local read "baud rate"() -> (w353:u32)
            n205 = Number To Decimal String(number=w353) -> (decimal integer string=w352:string)  [unwired: 1 in]
          }
        }
        n206 = feedback #1(w318) -> (w319:string)
        n207 = feedback-in #1(w318) -> ()
        n208 = case shown="\"2017-212协议\"" w326 {
          tunnel: ["32" ("设备编码MN") w345] -> w325
          frame "2005-212协议", Default {
          }
          frame "2017-212协议" {
            n209 = global read "断电保存全局.vi" "系统编码选择框"() -> (w346:string)
            n210 = case shown="\"污水排放过程监测\"" w346 {
              tunnel: ["52" ("设备编码MN") "32" ("设备编码MN") "21" ("设备编码MN")] -> w345
              frame "污水排放过程监测" {
              }
              frame "地表水体污染源" {
              }
              frame "地表水质量监测", Default {
              }
            }
          }
        }
        n211 = Not Equal?(x=w318, y=w319) -> (x != y?=w317:bool)
        n212 = Get Date/Time In Seconds() -> (seconds since 1Jan1904=w327:timestamp)
        n213 = feedback #2(w301) -> (w303:timestamp)
        n214 = feedback-in #2(w301) -> ()
        n215 = case shown="真" w317 {
          tunnel: w318 -> [_ w343]
          frame False {
          }
          frame True {
            n216 = global write "全局1.vi" "发送报文显示"(w343) -> ()
          }
        }
        n217 = Format Date/Time String(time format string (%c)="%Y/%m/%d %H:%M:%S" ("时间格式字符串(%c)"), seconds (now)=w327) -> (date/time string=→"系统时间":string)  [unwired: 1 in]
        n218 = Select(t=T14."Enabled" ("禁用"), s="更改起始时间", f=T14."Disabled and Grayed Out" ("禁用")) -> (s? t:f=w313:T14)
        n219 = Not Equal?(x=w301, y=w303) -> (x != y?=w302:bool)
        n220 = property on="数据发送起始时间" class="AbsTime (严格)"("DisabledEnum"=w313) -> ()  [unwired: 2 in, 2 out]
        n221 = property on="确定更改起始时间" class="Bool"("DisabledEnum"=w313) -> ()  [unwired: 2 in, 2 out]
        n222 = case shown="真" w302 {
          tunnel: w301 -> [_ w338]
          frame False {
          }
          frame True {
            n223 = local write "数据发送起始时间"(w338) -> ()
          }
        }
        n224 = global read "断电保存全局.vi" "配置表格"() -> (w299:string[][])
        n225 = local read "站点名称"() -> (w333:string)
        n226 = local read "站点设备"() -> (w332:string)
        n227 = Index Array(array=w299, index (col)=1 ("禁用的索引 (列)")) -> (element=w297:string[])  [unwired: 1 in]
        n228 = local read "MN"() -> (w330:string)
        n229 = local read "PW"() -> (w329:string)
        n230 = Array To Cluster(array=w297) -> (cluster=w300:T15)
        n231 = global write "断电保存全局.vi" "因子编码簇"(w300) -> ()
        n232 = global write "全局1.vi" "系统编码ST"(w325) -> ()
        n233 = Bundle By Name(cluster=T6 {"站点"="", "设备"="", "IP"="", "PORT"="", "MN"="", "PW"=""} ("配置信息"), "站点"=w333, "设备"=w332, "IP"=w334, "PORT"=w331, "MN"=w330, "PW"=w329) -> (→"配置信息":T6)
      }
    }
    n234 = Wait (ms)(milliseconds to wait=u32 1000 ("等待时间（毫秒）")) -> ()  [unwired: 1 out]
  }
  n235 = vi-ref "数据主动和反控发送.vi"() -> (w49:refnum<vi>)
  n236 = vi-ref "数采仪日志报警存储(子VI).vi"() -> (w50:refnum<vi>)
  n237 = while {
    stop <- FALSE stop-if-true
    n238 = event shown="[7] \"确定更改起始时间\": 值改变" {
      selector: _ -> [_ _ _ _ _ _ _ _ _ _ _ _]
      dyn-events: _ -> [_ _ _ _ _ _ _ _ _ _ _ _]
      timeout: _ -> [_ _ _ _ _ _ _ _ _ _ _ _]
      event Timeout {
        n239 = event-data() -> ()  [unwired: 1 in, 3 out]
      }
      event "站点名称", "站点设备", "IP", "PORT", "MN", "PW", "VISA resource name", "baud rate", "系统编码选择框", "每周自动重发", "重发日期", "重发时间": Value Change {
        n240 = event-data() -> ()  [unwired: 1 in, 6 out]
        n241 = flat-sequence {
          frame #0 {
            n242 = global write "断电保存全局.vi" "PW"("PW") -> ()
            n243 = global write "断电保存全局.vi" "站点名称"("站点名称") -> ()
            n244 = global write "断电保存全局.vi" "MN"("MN") -> ()
            n245 = global write "断电保存全局.vi" "PORT"("PORT") -> ()
            n246 = global write "断电保存全局.vi" "IP"("IP") -> ()
            n247 = global write "断电保存全局.vi" "重发日期"("重发日期") -> ()
            n248 = global write "断电保存全局.vi" "重发时间"("重发时间") -> ()
            n249 = global write "断电保存全局.vi" "站点设备"("站点设备") -> ()
            n250 = global write "断电保存全局.vi" "baud rate"("baud rate") -> ()
            n251 = global write "断电保存全局.vi" "系统编码选择框"("系统编码选择框") -> ()
            n252 = global write "断电保存全局.vi" "每周自动重发"("每周自动重发") -> ()
            n253 = global write "断电保存全局.vi" "VISA resource name"("VISA resource name") -> ()
          }
          frame #1 {
            n254 = call "配置文件断电保存(子VI).vi"() -> ()  [unwired: 12 in]
          }
        }
      }
      event "数据发送通道", "数据发送协议", "数据组合发送", "2011发送", "日志、参数发送", "判断数据反馈": Value Change {
        n255 = event-data() -> ("CtlRef"=w390:refnum<vi>, "OldVal"=w388:variant, "NewVal"=w387:variant)  [unwired: 1 in, 3 out]
        n256 = property class="Ctl"(reference=w390) -> ("Label.Text"=w389:string)  [unwired: 1 in, 2 out]
        n257 = case shown="\"数据发送协议\"" w389 {
          tunnel: w388 -> [_ w394 w417 w426 w449 w472 w495]
          tunnel: w387 -> [_ w391 w414 w423 w446 w469 w492]
          frame "假", Default {
          }
          frame "数据发送通道" {
            n258 = Variant To Data(type=enum16{"TCP", "VISA"}."TCP" ("数据发送通道"), Variant=w391) -> (data=w392:enum16{"TCP", "VISA"})  [unwired: 1 in, 1 out]
            n259 = global write "断电保存全局.vi" "数据发送通道"(w392) -> ()
            n260 = Two Button Dialog(message="TCP通过网络发送数据，VISA通过串口发送数据，确定更改数据发送通道吗？" ("消息")) -> (T button?=w395:bool)  [unwired: 2 in]
            n261 = case shown="假" w395 {
              tunnel: w394 -> [w398 _]
              frame False {
                n262 = Variant To Data(type=enum16{"TCP", "VISA"}."TCP" ("数据发送通道"), Variant=w398) -> (data=w397:enum16{"TCP", "VISA"})  [unwired: 1 in, 1 out]
                n263 = global write "断电保存全局.vi" "数据发送通道"(w397) -> ()
              }
              frame True {
                n264 = flat-sequence {
                  frame #0 {
                  }
                  frame #1 {
                    n265 = call <vilib>:"Application Directory.vi"() -> ("Application Directory"=w400:path)
                    n266 = Build Path(base path=w400, name or relative path="data\\sys.ini" ("名称或相对路径")) -> (appended path=w402:path)
                    n267 = call <vilib>:"Open Config Data.vi"("configuration file path"=w402) -> ("error out"=w406:errorcluster, "refnum"=w403:T11)  [unwired: 8 in, 1 out]
                    n268 = vi-ref "断电保存全局.vi"() -> (w404:refnum<vi>)
                    n269 = call <userlib>:"Write Panel to INI__ogtk.vi"("error in (no error)"=w406, "VI ref"=w404, "refnum"=w403) -> ("error out"=w407:errorcluster, "refnum out"=w405:T11)  [unwired: 7 in]
                    n270 = call <vilib>:"Close Config Data.vi"("error in (no error)"=w407, "refnum"=w405) -> ("error out"=w412:errorcluster, "file path"=w413:path)  [unwired: 8 in]
                    n271 = Open/Create/Replace File(file path (use dialog)=w413, error in=w412) -> (refnum out=w409:refnum<file>, error out=w408:errorcluster)  [unwired: 4 in, 1 out]
                    n272 = Flush File(refnum=w409, error in=w408) -> (refnum out=w410:refnum<file>, error out=w411:errorcluster)
                    n273 = Close File(refnum=w410, error in=w411) -> ()  [unwired: 2 out]
                  }
                }
              }
            }
          }
          frame "数据发送协议" {
            n274 = Variant To Data(type=enum16{"2005-212协议", "2017-212协议"}."2017-212协议" ("数据"), Variant=w414) -> (data=w415:enum16{"2005-212协议", "2017-212协议"})  [unwired: 1 in, 1 out]
            n275 = global write "断电保存全局.vi" "数据发送协议"(w415) -> ()
            n276 = Two Button Dialog(message="2005对应旧版通信协议，2017对应最新版协议，对应协议因子编码会不同，\n更改可能导致数据不能被平台识别，确定更改数据发送协议吗？" ("消息")) -> (T button?=w418:bool)  [unwired: 2 in]
            n277 = case shown="真" w418 {
              tunnel: w417 -> [w422 _]
              frame False {
                n278 = Variant To Data(type=enum16{"2005-212协议", "2017-212协议"}."2017-212协议" ("数据"), Variant=w422) -> (data=w420:enum16{"2005-212协议", "2017-212协议"})  [unwired: 1 in, 1 out]
                n279 = global write "断电保存全局.vi" "数据发送协议"(w420) -> ()
              }
              frame True {
                n280 = call "配置文件断电保存(子VI).vi"() -> ()  [unwired: 12 in]
              }
            }
          }
          frame "数据组合发送" {
            n281 = Variant To Data(type=FALSE, Variant=w423) -> (data=w424:bool)  [unwired: 1 in, 1 out]
            n282 = global write "断电保存全局.vi" "数据组合发送"(w424) -> ()
            n283 = Two Button Dialog(message="勾选数据组合发送功能表示所有参数打包整点同时上传、则只能整点发送延时较高，\n不勾选则表示单参数分别上传、则实时性较好，确定更改数据组合发送功能吗？" ("消息")) -> (T button?=w427:bool)  [unwired: 2 in]
            n284 = case shown="真" w427 {
              tunnel: w426 -> [w430 _]
              frame False {
                n285 = Variant To Data(type=FALSE, Variant=w430) -> (data=w429:bool)  [unwired: 1 in, 1 out]
                n286 = global write "断电保存全局.vi" "数据组合发送"(w429) -> ()
              }
              frame True {
                n287 = flat-sequence {
                  frame #0 {
                  }
                  frame #1 {
                    n288 = call <vilib>:"Application Directory.vi"() -> ("Application Directory"=w432:path)
                    n289 = Build Path(base path=w432, name or relative path="data\\sys.ini" ("名称或相对路径")) -> (appended path=w434:path)
                    n290 = call <vilib>:"Open Config Data.vi"("configuration file path"=w434) -> ("error out"=w438:errorcluster, "refnum"=w435:T11)  [unwired: 8 in, 1 out]
                    n291 = vi-ref "断电保存全局.vi"() -> (w436:refnum<vi>)
                    n292 = call <userlib>:"Write Panel to INI__ogtk.vi"("error in (no error)"=w438, "VI ref"=w436, "refnum"=w435) -> ("error out"=w439:errorcluster, "refnum out"=w437:T11)  [unwired: 7 in]
                    n293 = call <vilib>:"Close Config Data.vi"("error in (no error)"=w439, "refnum"=w437) -> ("error out"=w444:errorcluster, "file path"=w445:path)  [unwired: 8 in]
                    n294 = Open/Create/Replace File(file path (use dialog)=w445, error in=w444) -> (refnum out=w441:refnum<file>, error out=w440:errorcluster)  [unwired: 4 in, 1 out]
                    n295 = Flush File(refnum=w441, error in=w440) -> (refnum out=w442:refnum<file>, error out=w443:errorcluster)
                    n296 = Close File(refnum=w442, error in=w443) -> ()  [unwired: 2 out]
                  }
                }
              }
            }
          }
          frame "2011发送" {
            n297 = Variant To Data(type=FALSE, Variant=w446) -> (data=w447:bool)  [unwired: 1 in, 1 out]
            n298 = global write "断电保存全局.vi" "2011发送"(w447) -> ()
            n299 = Two Button Dialog(message="2011表示实时数据上传，一般情况需要勾选，确定更改2011实时数据发送功能吗？" ("消息")) -> (T button?=w450:bool)  [unwired: 2 in]
            n300 = case shown="真" w450 {
              tunnel: w449 -> [w453 _]
              frame False {
                n301 = Variant To Data(type=FALSE, Variant=w453) -> (data=w452:bool)  [unwired: 1 in, 1 out]
                n302 = global write "断电保存全局.vi" "2011发送"(w452) -> ()
              }
              frame True {
                n303 = flat-sequence {
                  frame #0 {
                  }
                  frame #1 {
                    n304 = call <vilib>:"Application Directory.vi"() -> ("Application Directory"=w455:path)
                    n305 = Build Path(base path=w455, name or relative path="data\\sys.ini" ("名称或相对路径")) -> (appended path=w457:path)
                    n306 = call <vilib>:"Open Config Data.vi"("configuration file path"=w457) -> ("error out"=w461:errorcluster, "refnum"=w458:T11)  [unwired: 8 in, 1 out]
                    n307 = vi-ref "断电保存全局.vi"() -> (w459:refnum<vi>)
                    n308 = call <userlib>:"Write Panel to INI__ogtk.vi"("error in (no error)"=w461, "VI ref"=w459, "refnum"=w458) -> ("error out"=w462:errorcluster, "refnum out"=w460:T11)  [unwired: 7 in]
                    n309 = call <vilib>:"Close Config Data.vi"("error in (no error)"=w462, "refnum"=w460) -> ("error out"=w467:errorcluster, "file path"=w468:path)  [unwired: 8 in]
                    n310 = Open/Create/Replace File(file path (use dialog)=w468, error in=w467) -> (refnum out=w464:refnum<file>, error out=w463:errorcluster)  [unwired: 4 in, 1 out]
                    n311 = Flush File(refnum=w464, error in=w463) -> (refnum out=w465:refnum<file>, error out=w466:errorcluster)
                    n312 = Close File(refnum=w465, error in=w466) -> ()  [unwired: 2 out]
                  }
                }
              }
            }
          }
          frame "日志、参数发送" {
            n313 = Variant To Data(type=FALSE, Variant=w469) -> (data=w470:bool)  [unwired: 1 in, 1 out]
            n314 = global write "断电保存全局.vi" "日志、参数发送"(w470) -> ()
            n315 = Two Button Dialog(message="选择是否需要仪器日志、状态和告警信息上传，一般情况需要勾选，确定更改日志、参数发送功能吗？" ("消息")) -> (T button?=w473:bool)  [unwired: 2 in]
            n316 = case shown="真" w473 {
              tunnel: w472 -> [w476 _]
              frame False {
                n317 = Variant To Data(type=FALSE, Variant=w476) -> (data=w475:bool)  [unwired: 1 in, 1 out]
                n318 = global write "断电保存全局.vi" "日志、参数发送"(w475) -> ()
              }
              frame True {
                n319 = flat-sequence {
                  frame #0 {
                  }
                  frame #1 {
                    n320 = call <vilib>:"Application Directory.vi"() -> ("Application Directory"=w478:path)
                    n321 = Build Path(base path=w478, name or relative path="data\\sys.ini" ("名称或相对路径")) -> (appended path=w480:path)
                    n322 = call <vilib>:"Open Config Data.vi"("configuration file path"=w480) -> ("error out"=w484:errorcluster, "refnum"=w481:T11)  [unwired: 8 in, 1 out]
                    n323 = vi-ref "断电保存全局.vi"() -> (w482:refnum<vi>)
                    n324 = call <userlib>:"Write Panel to INI__ogtk.vi"("error in (no error)"=w484, "VI ref"=w482, "refnum"=w481) -> ("error out"=w485:errorcluster, "refnum out"=w483:T11)  [unwired: 7 in]
                    n325 = call <vilib>:"Close Config Data.vi"("error in (no error)"=w485, "refnum"=w483) -> ("error out"=w490:errorcluster, "file path"=w491:path)  [unwired: 8 in]
                    n326 = Open/Create/Replace File(file path (use dialog)=w491, error in=w490) -> (refnum out=w487:refnum<file>, error out=w486:errorcluster)  [unwired: 4 in, 1 out]
                    n327 = Flush File(refnum=w487, error in=w486) -> (refnum out=w488:refnum<file>, error out=w489:errorcluster)
                    n328 = Close File(refnum=w488, error in=w489) -> ()  [unwired: 2 out]
                  }
                }
              }
            }
          }
          frame "判断数据反馈" {
            n329 = Variant To Data(type=FALSE, Variant=w492) -> (data=w493:bool)  [unwired: 1 in, 1 out]
            n330 = global write "断电保存全局.vi" "判断数据反馈"(w493) -> ()
            n331 = Two Button Dialog(message="勾选判断数据反馈是针对平台能有反馈的情况、此功能能保证数据的完整性，尽可能的防止各种问题导致的数据缺失，\n不勾选则表示数据只发送不判断平台的反馈、用于针对平台没有反馈的情况，确定更改判断数据反馈功能吗？" ("消息")) -> (T button?=w496:bool)  [unwired: 2 in]
            n332 = case shown="真" w496 {
              tunnel: w495 -> [w499 _]
              frame False {
                n333 = Variant To Data(type=FALSE, Variant=w499) -> (data=w498:bool)  [unwired: 1 in, 1 out]
                n334 = global write "断电保存全局.vi" "判断数据反馈"(w498) -> ()
              }
              frame True {
                n335 = flat-sequence {
                  frame #0 {
                  }
                  frame #1 {
                    n336 = call <vilib>:"Application Directory.vi"() -> ("Application Directory"=w501:path)
                    n337 = Build Path(base path=w501, name or relative path="data\\sys.ini" ("名称或相对路径")) -> (appended path=w503:path)
                    n338 = call <vilib>:"Open Config Data.vi"("configuration file path"=w503) -> ("error out"=w507:errorcluster, "refnum"=w504:T11)  [unwired: 8 in, 1 out]
                    n339 = vi-ref "断电保存全局.vi"() -> (w505:refnum<vi>)
                    n340 = call <userlib>:"Write Panel to INI__ogtk.vi"("error in (no error)"=w507, "VI ref"=w505, "refnum"=w504) -> ("error out"=w508:errorcluster, "refnum out"=w506:T11)  [unwired: 7 in]
                    n341 = call <vilib>:"Close Config Data.vi"("error in (no error)"=w508, "refnum"=w506) -> ("error out"=w513:errorcluster, "file path"=w514:path)  [unwired: 8 in]
                    n342 = Open/Create/Replace File(file path (use dialog)=w514, error in=w513) -> (refnum out=w510:refnum<file>, error out=w509:errorcluster)  [unwired: 4 in, 1 out]
                    n343 = Flush File(refnum=w510, error in=w509) -> (refnum out=w511:refnum<file>, error out=w512:errorcluster)
                    n344 = Close File(refnum=w511, error in=w512) -> ()  [unwired: 2 out]
                  }
                }
              }
            }
          }
        }
      }
      event "确定": Value Change {
        n345 = event-data() -> ()  [unwired: 1 in, 6 out]
        n346 = call "通信状态入队列.vi"("枚举"=enum16{"打开连接", "发送数据", "读取数据", "数据处理", "关闭连接"}."关闭连接") -> ()  [unwired: 10 in, 1 out]
      }
      event "配置表": Value Change {
        n347 = event-data() -> ()  [unwired: 1 in, 6 out]
        n348 = call "参数配置表.vi"() -> ()  [unwired: 12 in]
      }
      event "参数配置": Value Change {
        n349 = event-data() -> ()  [unwired: 1 in, 6 out]
        n350 = property on="窗格" class="Pane"("Origin"=T9 {"Horizontal"=0, "Vertical"=1000} ("原点")) -> ()  [unwired: 2 in, 2 out]
        n351 = call <vilib>:"Application Directory.vi"() -> ("Application Directory"=w517:path)
        n352 = call "查询启动项.vi"("启动文件路径"=w517) -> ("包含启动项"=w516:bool)  [unwired: 9 in, 1 out]
        n353 = local write "开机启动"(w516) -> ()
      }
      event "返回": Value Change {
        n354 = event-data() -> ()  [unwired: 1 in, 6 out]
        n355 = property on="窗格" class="Pane"("Origin"=T9 {"Horizontal"=0, "Vertical"=0} ("原点")) -> ()  [unwired: 2 in, 2 out]
      }
      event "确定更改起始时间": Value Change {
        n356 = event-data() -> ()  [unwired: 1 in, 6 out]
        n357 = local write "更改起始时间"(FALSE ("更改起始时间")) -> ()
        n358 = Two Button Dialog(message="确定以当前设置时间作为数据索引起始时间？" ("消息")) -> (T button?=w520:bool)  [unwired: 2 in]
        n359 = case shown="真" w520 {
          frame False {
          }
          frame True {
            n360 = global write "断电保存全局.vi" "数据重发"(TRUE ("数据重发")) -> ()
            n361 = Format Date/Time String(time format string (%c)="%Y/%m/%d %H:%M:%S" ("时间格式字符串(%c)"), seconds (now)="数据发送起始时间") -> (date/time string=w524:string)  [unwired: 1 in]
            n362 = global write "断电保存全局.vi" "数据重发时间戳"(w524) -> ()
            n363 = Initialize Array(w524, 31 ("维数大小")) -> (w525:string[])
            n364 = Array To Cluster(array=w525) -> (cluster=w523:T13)
            n365 = global write "全局 水样时间.vi" "水样数据索引"(w523) -> ()
            n366 = global read "断电保存全局.vi" "数据组合发送"() -> (w529:bool)
            n367 = case shown="假" w529 {
              tunnel: w524 -> [w531 _]
              frame False {
                n368 = global write "全局 时间2.vi" "标样核查索引起始时间"(w531) -> ()
                n369 = global write "全局 时间2.vi" "加标回收索引起始时间"(w531) -> ()
                n370 = global write "全局 时间2.vi" "跨度核查索引起始时间"(w531) -> ()
                n371 = global write "全局 时间2.vi" "零点核查索引起始时间"(w531) -> ()
                n372 = Initialize Array(w531, 8 ("维数大小")) -> (w537:string[])
                n373 = Initialize Array(w531, 15 ("维数大小")) -> (w532:string[])
                n374 = Array To Cluster(array=w537) -> (cluster=w536:T16)
                n375 = Array To Cluster(array=w532) -> (cluster=w533:T17)
                n376 = global write "全局 时间2.vi" "零点核查索引"(w536) -> ()
                n377 = global write "全局 时间2.vi" "跨度核查索引"(w536) -> ()
                n378 = global write "全局 时间2.vi" "标样核查索引"(w533) -> ()
                n379 = global write "全局 时间2.vi" "集成干预索引"(w533) -> ()
              }
              frame True {
              }
            }
          }
        }
      }
      event "开机启动": Value Change {
        n380 = event-data() -> ("CtlRef"=w539:refnum<vi>, "OldVal"=w538:bool, "NewVal"=w540:bool)  [unwired: 1 in, 3 out]
        n381 = case shown="真" w540 {
          tunnel: w539 -> [w542 w555]
          tunnel: w538 -> [w541 w554]
          frame False {
            n382 = Two Button Dialog(message="是否删除开机启动？" ("消息"), 1:"否" ("F按钮名称（“取消”）"), 2:"是" ("T按钮名称（“确定”）")) -> (T button?=w543:bool)
            n383 = case shown="假" w543 {
              tunnel: w542 -> [w548 _]
              tunnel: w541 -> [w547 _]
              frame False {
                n384 = property class="Bool (严格)"(reference=w548, "Value"=w547) -> ()  [unwired: 1 in, 2 out]
              }
              frame True {
                n385 = call <vilib>:"Application Directory.vi"() -> ("Application Directory"=w550:path)
                n386 = call "删除启动项.vi"("启动文件路径"=w550) -> ("删除标记"=w549:bool)  [unwired: 9 in, 1 out]
                n387 = case shown="假" w549 {
                  tunnel: ["删除开机启动失败" ("T按钮名称（“确定”）") "删除开机启动成功" ("T按钮名称（“确定”）")] -> w551
                  frame False {
                  }
                  frame True {
                  }
                }
                n388 = One Button Dialog(message=w551) -> ()  [unwired: 1 in, 1 out]
              }
            }
          }
          frame True {
            n389 = Two Button Dialog(message="是否添加开机启动？" ("消息"), 1:"否" ("F按钮名称（“取消”）"), 2:"是" ("T按钮名称（“确定”）")) -> (T button?=w556:bool)
            n390 = case shown="真" w556 {
              tunnel: w555 -> [w561 _]
              tunnel: w554 -> [w560 _]
              frame False {
                n391 = property class="Bool (严格)"(reference=w561, "Value"=w560) -> ()  [unwired: 1 in, 2 out]
              }
              frame True {
                n392 = call <vilib>:"Application Directory.vi"() -> ("Application Directory"=w564:path)
                n393 = call "添加启动项.vi"("启动文件路径"=w564) -> ("添加成功标记"=w563:bool)  [unwired: 9 in, 1 out]
                n394 = case shown="真" w563 {
                  tunnel: ["添加开机启动失败" ("T按钮名称（“确定”）") "添加开机启动成功" ("T按钮名称（“确定”）")] -> w562
                  frame False {
                  }
                  frame True {
                  }
                }
                n395 = One Button Dialog(message=w562) -> ()  [unwired: 1 in, 1 out]
              }
            }
          }
        }
      }
      event "更新": Value Change {
        n396 = event-data() -> ()  [unwired: 1 in, 6 out]
        n397 = call "自定义双按钮对话框.vi"("消息"="选择是否从服务器获取最新版本信息？") -> ("输出"=w567:bool)  [unwired: 10 in]
        n398 = case shown="真" w567 {
          frame False {
          }
          frame True {
            # "获取最新版本"
            n399 = call "FTP自动升级更新main.vi"() -> ()  [unwired: 12 in]
          }
        }
      }
      event "updateconfiguration": Value Change {
        n400 = event-data() -> ("NewVal"=w576:T2)  [unwired: 1 in, 5 out]
        n401 = call <vilib>:"Application Directory.vi"() -> ("Application Directory"=w580:path)
        n402 = Build Array("主机" ("section"), "用户" ("section"), "密码" ("key"), "远程路径" ("key"), "下载文件名" ("key"), "软件版本" ("key")) -> (w569:string[])
        n403 = Build Path(base path=w580, name or relative path="update\\data\\set.ini" ("名称或相对路径")) -> (appended path=w578:path)
        n404 = call "配置文件write.vi"("updateconfiguration"=w576, "configuration file path"=w578, "键数组"=w569, "段"="应用程序交互" ("section")) -> ("error out"=w577:errorcluster)  [unwired: 7 in]
        n405 = call <vilib>:"Clear Errors.vi"("error in (no error)"=w577) -> ()  [unwired: 5 in, 2 out]
      }
      event "IP", "PORT": Mouse Down {
        n406 = event-data() -> ("CtlRef"=w585:refnum<vi>)  [unwired: 1 in, 7 out]
        n407 = property class="Str"(reference=w585) -> (reference out=w583:refnum<vi>, "Value"=w584:string)  [unwired: 1 in, 1 out]
        n408 = call "IP键盘.vi"("OldNumber"=w584) -> ("NewNumber"=w582:string)
        n409 = property class="Str"(reference=w583, "Val(Sgnl)"=w582) -> ()  [unwired: 1 in, 2 out]
      }
    }
  }
  n410 = Obtain Queue(name (unnamed)="actualwrite" ("名称（未命名）"), element data type=enum16{"打开连接", "发送数据", "读取数据", "数据处理", "关闭连接"}."打开连接" ("枚举")) -> (queue out=w37:refnum<queue>, error out=w36:errorcluster)  [unwired: 3 in, 1 out]
  n411 = Obtain Queue(name (unnamed)="actualread" ("名称（未命名）"), element data type=enum16{"打开连接", "发送数据", "读取数据", "数据处理", "关闭连接"}."打开连接" ("枚举")) -> (queue out=w34:refnum<queue>, error out=w27:errorcluster)  [unwired: 3 in, 1 out]
  n412 = property class="VI"(reference=w49) -> ("Name"=w48:string)  [unwired: 1 in, 2 out]
  n413 = property class="VI"(reference=w50) -> ("Name"=w57:string)  [unwired: 1 in, 2 out]
  n414 = while {
    tunnel: w37 -> [w594]
    tunnel: w36 -> [w593]
    shift-right: [w589] -> _
    shift-left: errorcluster {"status"=FALSE, "code"=0, "source"=""} ("error out") -> [w588]
    stop <- FALSE stop-if-true
    # "写入数据出队列"
    n415 = Dequeue Element(queue=w594, timeout in ms (-1)=30000 ("超时毫秒(-1)"), error in (no error)=w593) -> (queue out=w587:refnum<queue>, element=w591:enum16{"打开连接", "发送数据", "读取数据", "数据处理", "关闭连接"}, timed out?=w590:bool, error out=w586:errorcluster)
    n416 = case shown="无错误" w588 {
      tunnel: w591 -> [w596 _]
      tunnel: w590 -> [w598 _]
      tunnel: [w602 w643] -> w589
      tunnel: w588 -> [w601 w647]
      tunnel: w587 -> [w600 w645]
      tunnel: w586 -> [w599 w644]
      frame No Error {
        n417 = case shown="真" w598 {
          tunnel: [w603 enum16{"打开连接", "发送数据", "读取数据", "数据处理", "关闭连接"}."发送数据" ("枚举")] -> w597
          tunnel: w596 -> [w603 _]
          frame False {
          }
          frame True {
          }
        }
        n418 = case shown="\"发送数据\", 默认" w597 {
          tunnel: w598 -> [_ w620 _ _ _]
          tunnel: [w606 w615 _ _ w636] -> w602
          tunnel: w601 -> [w608 w622 _ _ w637]
          tunnel: w600 -> [_ _ _ _ w638]
          tunnel: w599 -> [_ _ _ _ w635]
          frame "打开连接" {
            n419 = global read "断电保存全局.vi" "VISA resource name"() -> (w614:refnum<visa-resource-name>)
            n420 = global read "断电保存全局.vi" "数据发送通道"() -> (w611:enum16{"TCP", "VISA"})
            n421 = global read "断电保存全局.vi" "baud rate"() -> (w613:u32)
            n422 = global read "断电保存全局.vi" "PORT"() -> (w612:string)
            n423 = global read "断电保存全局.vi" "IP"() -> (w610:string)
            n424 = call "VISATCP组合选择发送.vi"("IP"=w610, "数据发送通道"=w611, "命令"="open", "PORT"=w612, "VISA resource name"=w614, "baud rate"=w613, "error in (no error)"=w608) -> ("错误输出"=w606:errorcluster)  [unwired: 5 in, 3 out]
            n425 = Unbundle By Name(w606) -> ("status"=w605:bool)  [unwired: 1 out]
            n426 = Not(x=w605) -> (.not. x?=w607:bool)
            n427 = global write "全局 数据发送重叠.vi" "掉线指示灯"(w605) -> ()
            n428 = local write "通信状态"(w607) -> ()
          }
          frame "发送数据", Default {
            n429 = case shown="真" w620 {
              tunnel: [w627 w629] -> w617
              tunnel: w622 -> [w626 w630]
              tunnel: [w626 w630] -> w621
              frame False {
                # "事件触发发送数据"
                n430 = global read "全局1.vi" "发送报文显示"() -> (w627:string)
              }
              frame True {
                # "30秒超时发送心跳包"
                n431 = local read "配置信息"() -> (w633:T6)
                n432 = Unbundle By Name(w633) -> ("MN"=w632:string, "PW"=w631:string)
                n433 = call "数据编码.vi"("table输入"="心跳包", "MN"=w632, "PW"=w631) -> ("通讯包字符串"=w629:string)  [unwired: 11 in, 1 out]
                n434 = global write "全局1.vi" "发送报文显示"(w629) -> ()
                n435 = Wait (ms)(milliseconds to wait=u32 500 ("等待时间（毫秒）")) -> ()  [unwired: 1 out]
              }
            }
            n436 = global read "断电保存全局.vi" "数据发送通道"() -> (w623:enum16{"TCP", "VISA"})
            n437 = Concatenate Strings("send:" ("字符串"), w617) -> (w616:string)
            n438 = call "VISATCP组合选择发送.vi"("数据发送通道"=w623, "命令"="write", "error in (no error)"=w621, "写入缓冲区"=w617) -> ("错误输出"=w615:errorcluster)  [unwired: 8 in, 3 out]
            n439 = Build Array(w616) -> (w619:string[])
            n440 = call "发送数据记录到文档(子VI).vi"("数组"=w619) -> ()  [unwired: 9 in, 1 out]
            n441 = flat-sequence {
              tunnel: w615 -> [_]
              frame #0 {
                n442 = local write "心跳包"(FALSE ("心跳包")) -> ()
              }
            }
            "心跳包" <- w620
          }
          frame "读取数据" {
          }
          frame "数据处理" {
          }
          frame "关闭连接" {
            n443 = global read "断电保存全局.vi" "数据发送通道"() -> (w640:enum16{"TCP", "VISA"})
            n444 = Enqueue Element(queue=w638, element=enum16{"打开连接", "发送数据", "读取数据", "数据处理", "关闭连接"}."打开连接" ("枚举"), error in (no error)=w635) -> ()  [unwired: 1 in, 3 out]
            n445 = call "VISATCP组合选择发送.vi"("数据发送通道"=w640, "命令"="close", "error in (no error)"=w637) -> ("错误输出"=w641:errorcluster)  [unwired: 9 in, 3 out]
            n446 = call <vilib>:"Clear Errors.vi"("error in (no error)"=w641) -> ("error out"=w636:errorcluster)  [unwired: 5 in, 1 out]
          }
        }
      }
      frame Error {
        n447 = Unbundle By Name(w647) -> ("code"=w646:i32)
        n448 = case shown="0, 默认" w646 {
          tunnel: w645 -> [w654 w670 w682]
          tunnel: w644 -> [w653 w669 w681]
          tunnel: [w652 w667 w680] -> w643
          frame 0, Default {
            n449 = Flush Queue(queue=w654, error in (no error)=w653) -> (queue out=w656:refnum<queue>, error out=w657:errorcluster)  [unwired: 1 out]
            n450 = local read "状态信息"() -> (w651:T5)
            n451 = Unbundle By Name(w651) -> ("TCP服务端掉线计数"=w649:i32)
            n452 = Enqueue Element(queue=w656, element=enum16{"打开连接", "发送数据", "读取数据", "数据处理", "关闭连接"}."关闭连接" ("枚举"), error in (no error)=w657) -> (error out=w658:errorcluster)  [unwired: 1 in, 2 out]
            n453 = Increment(x=w649) -> (x+1=w650:i32)
            n454 = Bundle By Name(cluster=w651, "TCP服务端掉线计数"=w650) -> (w648:T5)
            n455 = local write "状态信息"(w648) -> ()
            n456 = call <vilib>:"Clear Errors.vi"("error in (no error)"=w658) -> ("error out"=w652:errorcluster)  [unwired: 5 in, 1 out]
          }
          frame 54, 63 {
            n457 = Flush Queue(queue=w670, error in (no error)=w669) -> (queue out=w672:refnum<queue>, error out=w673:errorcluster)  [unwired: 1 out]
            n458 = local read "状态信息"() -> (w662:T5)
            n459 = Unbundle By Name(w662) -> ("TCP服务端掉线计数"=w666:i32, "TCP掉线时间节点"=w659:string)
            n460 = Enqueue Element(queue=w672, element=enum16{"打开连接", "发送数据", "读取数据", "数据处理", "关闭连接"}."关闭连接" ("枚举"), error in (no error)=w673) -> (error out=w668:errorcluster)  [unwired: 1 in, 2 out]
            n461 = Less Or Equal?(x=w666, y=1) -> (x <= y?=w664:bool)
            n462 = case shown="真" w664 {
              tunnel: [w674 w675] -> w663
              tunnel: w659 -> [w674 _]
              frame False {
              }
              frame True {
                n463 = Get Date/Time In Seconds() -> (seconds since 1Jan1904=w676:timestamp)
                n464 = Format Date/Time String(time format string (%c)="%Y%m%d%H%M%S%3u" ("时间格式字符串(%c)"), seconds (now)=w676) -> (date/time string=w678:string)  [unwired: 1 in]
                n465 = call "格式时间字符串.vi"("字符串"=w678) -> ("连接的字符串"=w675:string)  [unwired: 10 in]
              }
            }
            n466 = Increment(x=w666) -> (x+1=w661:i32)
            n467 = call <vilib>:"Clear Errors.vi"("error in (no error)"=w668) -> ("error out"=w667:errorcluster)  [unwired: 5 in, 1 out]
            n468 = Bundle By Name(cluster=w662, "TCP服务端掉线计数"=w661, "TCP掉线时间节点"=w663) -> (w660:T5)
            n469 = local write "状态信息"(w660) -> ()
          }
          frame 56 {
            n470 = Flush Queue(queue=w682, error in (no error)=w681) -> (error out=w679:errorcluster)  [unwired: 2 out]
            n471 = call <vilib>:"Clear Errors.vi"("error in (no error)"=w679) -> ("error out"=w680:errorcluster)  [unwired: 5 in, 1 out]
          }
        }
      }
    }
  }
  n472 = call <vilib>:"Application Directory.vi"() -> ("Application Directory"=w64:path)
  n473 = property class="App"() -> ("App.Name"=w4:string)  [unwired: 2 in, 2 out]
  n474 = Open VI Reference(type specifier VI Refnum (for type only)=refnum<vi> refnum, vi path=w48, options=128 ("选项")) -> (vi reference=w46:refnum<vi>, error out=w44:errorcluster)  [unwired: 3 in]
  n475 = Open VI Reference(type specifier VI Refnum (for type only)=refnum<vi> refnum, vi path=w57, options=128 ("选项")) -> (vi reference=w55:refnum<vi>, error out=w53:errorcluster)  [unwired: 3 in]
  n476 = Obtain Queue(name (unnamed)="反控命令信息队列" ("名称（未命名）"), element data type=cluster{"命令编码CN":string, "QN":string} {"命令编码CN"="", "QN"=""}) -> (queue out=w21:refnum<queue>, error out=w20:errorcluster)  [unwired: 3 in, 1 out]
  n477 = Build Path(base path=w64, name or relative path="data\\tubiao.ico" ("名称或相对路径")) -> (appended path=w72:path)
  n478 = Enqueue Element(queue=w34, element=enum16{"打开连接", "发送数据", "读取数据", "数据处理", "关闭连接"}."打开连接" ("枚举"), error in (no error)=w27) -> (queue out=w30:refnum<queue>, error out=w29:errorcluster)  [unwired: 1 in, 1 out]
  n479 = Obtain Queue(name (unnamed)="datasent" ("名称（未命名）"), element data type="实时小时数据" ("元素")) -> (queue out=w25:refnum<queue>, error out=w24:errorcluster)  [unwired: 3 in, 1 out]
  n480 = Current VI's Path() -> (path=w61:path)
  n481 = call-by-ref "?"(reference=w46, error in=w44) -> (reference out=w42:refnum<vi>, error out=w43:errorcluster)  [unwired: 12 in]
  n482 = call-by-ref "?"(reference=w55, error in=w53) -> (reference out=w51:refnum<vi>, error out=w52:errorcluster)  [unwired: 12 in]
  n483 = Build Array(w72) -> (w67:path[])
  n484 = Open VI Reference(vi path=w61) -> (vi reference=w60:refnum<vi>)  [unwired: 5 in, 1 out]
  n485 = Close Reference(reference=w42, error in (no error)=w43) -> ()  [unwired: 1 out]
  n486 = Close Reference(reference=w51, error in (no error)=w52) -> ()  [unwired: 1 out]
  n487 = invoke class="VI" method="FP.Open"(reference=w60, "Activate"=TRUE ("激活？"), "State"=T7."Standard" ("状态")) -> (error out=w59:errorcluster)  [unwired: 2 in, 4 out]
  n488 = while {
    tunnel: w30 -> [w695]
    tunnel: w29 -> [w694]
    shift-right: [w691] -> _
    shift-left: errorcluster {"status"=FALSE, "code"=0, "source"=""} ("error out") -> [w690]
    tunnel: w25 -> [w686]
    tunnel: w24 -> [w685]
    tunnel: w21 -> [w684]
    tunnel: w20 -> [w683]
    stop <- FALSE stop-if-true
    # "读取数据出队列处理"
    n489 = Dequeue Element(queue=w695, error in (no error)=w694) -> (queue out=w689:refnum<queue>, element=w692:enum16{"打开连接", "发送数据", "读取数据", "数据处理", "关闭连接"}, error out=w688:errorcluster)  [unwired: 1 in, 1 out]
    n490 = Wait (ms)(milliseconds to wait=u32 1000 ("等待时间（毫秒）")) -> ()  [unwired: 1 out]
    n491 = case shown="无错误" w690 {
      tunnel: w692 -> [w701 _]
      tunnel: [w708 w786] -> w691
      tunnel: w690 -> [w707 w790]
      tunnel: w689 -> [w706 w788]
      tunnel: w688 -> [w705 w787]
      tunnel: w686 -> [w699 _]
      tunnel: w685 -> [w698 _]
      tunnel: w684 -> [w697 _]
      tunnel: w683 -> [w696 _]
      frame No Error {
        n492 = case shown="\"打开连接\", 默认" w701 {
          tunnel: [w715 _ w749 _ w781] -> w708
          tunnel: w707 -> [w714 _ w752 _ w782]
          tunnel: w706 -> [w712 _ w744 _ w779]
          tunnel: w705 -> [w711 _ w743 _ w778]
          tunnel: [w710 _ _ _ _] -> w702
          tunnel: w699 -> [_ _ w736 _ _]
          tunnel: w698 -> [_ _ w735 _ _]
          tunnel: w697 -> [_ _ w724 _ _]
          tunnel: w696 -> [_ _ w723 _ _]
          frame "打开连接", Default {
            n493 = Enqueue Element(queue=w712, element=enum16{"打开连接", "发送数据", "读取数据", "数据处理", "关闭连接"}."读取数据" ("枚举"), error in (no error)=w711) -> ()  [unwired: 1 in, 3 out]
            n494 = global read "断电保存全局.vi" "VISA resource name"() -> (w722:refnum<visa-resource-name>)
            n495 = global read "断电保存全局.vi" "数据发送通道"() -> (w719:enum16{"TCP", "VISA"})
            n496 = global read "断电保存全局.vi" "baud rate"() -> (w721:u32)
            n497 = global read "断电保存全局.vi" "PORT"() -> (w720:string)
            n498 = global read "断电保存全局.vi" "IP"() -> (w718:string)
            n499 = call "VISATCP组合选择发送.vi"("IP"=w718, "数据发送通道"=w719, "命令"="open", "PORT"=w720, "VISA resource name"=w722, "baud rate"=w721, "error in (no error)"=w714) -> ("错误输出"=w715:errorcluster)  [unwired: 5 in, 3 out]
            n500 = Unbundle By Name(w715) -> ("status"=w709:bool, "code"=w710:i32)
            n501 = Not(x=w709) -> (.not. x?=→"通信状态":bool)
            n502 = global write "全局 数据发送重叠.vi" "掉线指示灯"(w709) -> ()
          }
          frame "发送数据" {
          }
          frame "读取数据" {
            n503 = Get Queue Status(queue=w744, error in (no error)=w743) -> (queue out=w740:refnum<queue>, error out=w739:errorcluster, # elements in queue=w742:i32)  [unwired: 1 in, 5 out]
            n504 = global read "断电保存全局.vi" "数据发送通道"() -> (w751:enum16{"TCP", "VISA"})
            n505 = Equal To 0?(x=w742) -> (x = 0?=w741:bool)
            n506 = case shown="真" w741 {
              tunnel: w740 -> [_ w776]
              tunnel: w739 -> [_ w775]
              frame False {
              }
              frame True {
                n507 = Enqueue Element(queue=w776, element=enum16{"打开连接", "发送数据", "读取数据", "数据处理", "关闭连接"}."读取数据" ("枚举"), error in (no error)=w775) -> ()  [unwired: 1 in, 3 out]
              }
            }
            n508 = call "VISATCP组合选择发送.vi"("数据发送通道"=w751, "命令"="read", "error in (no error)"=w752) -> ("读取缓冲区"=w737:string, "错误输出"=w749:errorcluster)  [unwired: 9 in, 2 out]
            n509 = call "读取数据处理 (子VI).vi"("data out"=w737) -> ("命令编码CN"=w745:string, "数据"=w733:string, "时间QN"=w725:string)  [unwired: 8 in, 4 out]
            n510 = Empty String/Path?(string/path=w737) -> (empty?=w738:bool)
            n511 = case shown="假" w738 {
              tunnel: w737 -> [w772 _]
              tunnel: w725 -> [w769 _]
              frame False {
                n512 = Search/Split String(string=w769, search string/char (-)="QN=" ("搜索字符串/字符(-)")) -> (match + rest of string=w768:string)  [unwired: 1 in, 2 out]
                n513 = global write "全局1.vi" "数据输出"(w772) -> ()
                n514 = global write "全局1.vi" "读取报文显示"(w772) -> ()
                n515 = String Subset(string=w768, offset (0)=3 ("偏移量(0)")) -> (substring=w767:string)  [unwired: 1 in]
                n516 = global write "全局1.vi" "QN"(w767) -> ()
                n517 = call "数据记录.vi"("写入字段"=w772) -> ("连接的字符串"=w773:string)  [unwired: 10 in]
                n518 = Build Array(w773) -> (w774:string[])
                n519 = call "发送数据记录到文档(子VI).vi"("数组"=w774) -> ()  [unwired: 9 in, 1 out]
              }
              frame True {
              }
            }
            n520 = Search/Split String(string=w745, search string/char (-)="CN=" ("搜索字符串/字符(-)")) -> (match + rest of string=w746:string)  [unwired: 1 in, 2 out]
            n521 = String Subset(string=w746, offset (0)=3 ("偏移量(0)")) -> (substring=w731:string)  [unwired: 1 in]
            n522 = Empty String/Path?(string/path=w731) -> (empty?=w734:bool)
            n523 = Not Equal?(x=w731, y="9013") -> (x != y?=w728:bool)
            n524 = Not Equal?(x=w731, y="9014") -> (x != y?=w727:bool)
            n525 = Not(x=w734) -> (.not. x?=w726:bool)
            n526 = Compound Arithmetic op=AND ("复合运算")(w726, w728, w727) -> (w732:bool)
            n527 = case shown="真" w732 {
              tunnel: w736 -> [_ w766]
              tunnel: w735 -> [_ w765]
              tunnel: w733 -> [_ w764]
              tunnel: w731 -> [_ w755]
              tunnel: w725 -> [_ w760]
              tunnel: w724 -> [_ w759]
              tunnel: w723 -> [_ w758]
              frame False {
              }
              frame True {
                n528 = global write "全局1.vi" "数据"(w764) -> ()
                n529 = Search/Split String(string=w760, search string/char (-)="QN=" ("搜索字符串/字符(-)")) -> (match + rest of string=w763:string)  [unwired: 1 in, 2 out]
                n530 = global write "全局1.vi" "命令编码CN"(w755) -> ()
                n531 = String Subset(string=w763, offset (0)=3 ("偏移量(0)")) -> (substring=w754:string)  [unwired: 1 in]
                n532 = Bundle By Name(cluster=cluster{"命令编码CN":string, "QN":string} {"命令编码CN"="", "QN"=""}, "命令编码CN"=w755, "QN"=w754) -> (w756:cluster{"命令编码CN":string, "QN":string})
                n533 = Enqueue Element At Opposite End(queue=w766, element="反控命令" ("元素"), error in (no error)=w765) -> ()  [unwired: 1 in, 3 out]
                n534 = Enqueue Element(queue=w759, element=w756, error in (no error)=w758) -> ()  [unwired: 1 in, 3 out]
              }
            }
          }
          frame "数据处理" {
          }
          frame "关闭连接" {
            n535 = global read "断电保存全局.vi" "数据发送通道"() -> (w784:enum16{"TCP", "VISA"})
            n536 = Enqueue Element(queue=w779, element=enum16{"打开连接", "发送数据", "读取数据", "数据处理", "关闭连接"}."打开连接" ("枚举"), error in (no error)=w778) -> ()  [unwired: 1 in, 3 out]
            n537 = call "VISATCP组合选择发送.vi"("数据发送通道"=w784, "命令"="close", "error in (no error)"=w782) -> ("错误输出"=w783:errorcluster)  [unwired: 9 in, 3 out]
            n538 = call <vilib>:"Clear Errors.vi"("error in (no error)"=w783) -> ("error out"=w781:errorcluster)  [unwired: 5 in, 1 out]
          }
        }
        n539 = local read "状态信息"() -> (w704:T5)
        n540 = Bundle By Name(cluster=w704, "TCP服务端掉线计数"=0, "1st Error to Convert"=w702, "步骤"=w701) -> (→"状态信息":T5)
      }
      frame Error {
        n541 = Unbundle By Name(w790) -> ("code"=w789:i32)
        n542 = case shown="54, 63" w789 {
          tunnel: w788 -> [w797 w813 w824]
          tunnel: w787 -> [w796 w812 w823]
          tunnel: [w795 w810 w822] -> w786
          frame 0, Default {
            n543 = Flush Queue(queue=w797, error in (no error)=w796) -> (queue out=w799:refnum<queue>, error out=w800:errorcluster)  [unwired: 1 out]
            n544 = local read "状态信息"() -> (w794:T5)
            n545 = Enqueue Element(queue=w799, element=enum16{"打开连接", "发送数据", "读取数据", "数据处理", "关闭连接"}."关闭连接" ("枚举"), error in (no error)=w800) -> (error out=w801:errorcluster)  [unwired: 1 in, 2 out]
            n546 = Unbundle By Name(w794) -> ("TCP服务端掉线计数"=w792:i32)
            n547 = Increment(x=w792) -> (x+1=w793:i32)
            n548 = Bundle By Name(cluster=w794, "TCP服务端掉线计数"=w793) -> (w791:T5)
            n549 = local write "状态信息"(w791) -> ()
            n550 = call <vilib>:"Clear Errors.vi"("error in (no error)"=w801) -> ("error out"=w795:errorcluster)  [unwired: 5 in, 1 out]
          }
          frame 54, 63 {
            n551 = Flush Queue(queue=w813, error in (no error)=w812) -> (queue out=w815:refnum<queue>, error out=w816:errorcluster)  [unwired: 1 out]
            n552 = local read "状态信息"() -> (w805:T5)
            n553 = Unbundle By Name(w805) -> ("TCP服务端掉线计数"=w809:i32, "TCP掉线时间节点"=w802:string)
            n554 = Enqueue Element(queue=w815, element=enum16{"打开连接", "发送数据", "读取数据", "数据处理", "关闭连接"}."关闭连接" ("枚举"), error in (no error)=w816) -> (error out=w811:errorcluster)  [unwired: 1 in, 2 out]
            n555 = Less Or Equal?(x=w809, y=1) -> (x <= y?=w807:bool)
            n556 = Increment(x=w809) -> (x+1=w804:i32)
            n557 = case shown="真" w807 {
              tunnel: [w817 w818] -> w806
              tunnel: w802 -> [w817 _]
              frame False {
              }
              frame True {
                n558 = Get Date/Time In Seconds() -> (seconds since 1Jan1904=w819:timestamp)
                n559 = Format Date/Time String(time format string (%c)="%Y%m%d%H%M%S%3u" ("时间格式字符串(%c)"), seconds (now)=w819) -> (date/time string=w821:string)  [unwired: 1 in]
                n560 = call "格式时间字符串.vi"("字符串"=w821) -> ("连接的字符串"=w818:string)  [unwired: 10 in]
              }
            }
            n561 = call <vilib>:"Clear Errors.vi"("error in (no error)"=w811) -> ("error out"=w810:errorcluster)  [unwired: 5 in, 1 out]
            n562 = Bundle By Name(cluster=w805, "TCP服务端掉线计数"=w804, "TCP掉线时间节点"=w806) -> (w803:T5)
            n563 = local write "状态信息"(w803) -> ()
          }
          frame 56 {
            n564 = Flush Queue(queue=w824, error in (no error)=w823) -> (queue out=w826:refnum<queue>, error out=w827:errorcluster)  [unwired: 1 out]
            n565 = Enqueue Element(queue=w826, element=enum16{"打开连接", "发送数据", "读取数据", "数据处理", "关闭连接"}."读取数据" ("枚举"), error in (no error)=w827) -> (error out=w828:errorcluster)  [unwired: 1 in, 2 out]
            n566 = call <vilib>:"Clear Errors.vi"("error in (no error)"=w828) -> ("error out"=w822:errorcluster)  [unwired: 5 in, 1 out]
          }
        }
      }
    }
  }
  n567 = Build Array("Open", w4, "Exit" ("元素")) -> (w2:string[])
  n568 = call <vilib>:"Constructor.vi"("error in"=w59, "IconFilePathList"=w67) -> ("error out"=w71:errorcluster, "NotifyIcon"=w65:refnum<class "NotifyIcon.lvclass">)  [unwired: 8 in]
  n569 = for {
    shift-right: [w833] -> w83
    shift-left: w71 -> [w834]
    tunnel: w2 -> [w832] mode=indexing
    tunnel: w1 -> [w831] mode=indexing
    shift-right: [w829] -> w82
    shift-left: w65 -> [w830]
    # "2."
    n570 = call <vilib>:"InsertMenuItem.vi"("error in"=w834, "ItemTag"=w831, "ItemName"=w832, "NotifyIcon in"=w830) -> ("error out"=w833:errorcluster, "NotifyIcon out"=w829:refnum<class "NotifyIcon.lvclass">)  [unwired: 6 in]
  }
  n571 = Index Array(array=w1) -> (element=w66:string)  [unwired: 1 in]
  n572 = property class="NotifyIcon"(reference=w82, error in=w83, "Public:Visible"=TRUE ("Visible"), "Public:DefaultMenuItem"=w66, "Public:TipText"="平台数据传输系统" ("TipText")) -> (reference out=w79:refnum<class "NotifyIcon.lvclass">, error out=w70:errorcluster, "Public:SelectedItemEvent"=w69:refnum<user-event>)
  n573 = register-events(error in=w70, w69) -> (reference out=w40:refnum<event-registration>, error out=w41:errorcluster)  [unwired: 1 in]
  n574 = while {
    shift-right: [w838] -> w77
    shift-left: w41 -> [w837]
    shift-right: [w839] -> w74
    shift-left: w79 -> [w840]
    shift-right: [w836] -> w75
    shift-left: w40 -> [w841]
    tunnel: [w835] -> _
    stop <- w835 stop-if-true
    n575 = case shown="无错误" w837 {
      selector: w837 -> [w843 w874]
      tunnel: w841 -> [w848 w869]
      tunnel: w840 -> [w847 w870]
      tunnel: [w846 w870] -> w839
      tunnel: [w845 w872] -> w838
      tunnel: [w844 FALSE ("Discard?")] -> w835
      tunnel: [w842 w869] -> w836
      frame No Error {
        n576 = event shown="[1] 前面板关闭？" {
          selector: w848 -> [_ _]
          dyn-events: [_ _] -> w842
          timeout: _ -> [_ _]
          tunnel: w843 -> [w851 w867]
          tunnel: [w851 w866] -> w845
          tunnel: [w850 FALSE ("Discard?")] -> w844
          tunnel: w847 -> [w849 w868]
          tunnel: [w849 w865] -> w846
          event User Event {
            # "5."
            n577 = event-data() -> ("ItemTag"=w852:string)  [unwired: 1 in]
            n578 = case shown="默认" w852 {
              tunnel: [FALSE TRUE] -> w850
              frame Default {
                n579 = Current VI's Path() -> (path=w854:path)
                n580 = Open VI Reference(vi path=w854) -> (vi reference=w855:refnum<vi>)  [unwired: 5 in, 1 out]
                n581 = invoke class="VI" method="FP.Open"(reference=w855, "Activate"=TRUE ("激活？"), "State"=T7."Standard" ("状态")) -> ()  [unwired: 2 in, 5 out]
              }
              frame "EXIT" {
              }
            }
          }
          event Panel Close? {
            # "4."
            n582 = event-data() -> ("VIRef"=w861:refnum<vi>)  [unwired: 1 in, 3 out]
            n583 = invoke class="VI" method="FP.Open"(reference=w861, "State"=T7."Hidden" ("状态")) -> ()  [unwired: 3 in, 5 out]
            n584 = call <vilib>:"ShowBalloonTip.vi"("Balloon Icon"=BalloonIcon."Information", "error in"=w867, "Text"="欢迎使用平台数据传输系统", "NotifyIcon in"=w868) -> ("error out"=w866:errorcluster, "NotifyIcon out"=w865:refnum<class "NotifyIcon.lvclass">)  [unwired: 6 in]
            n585 = event-data("Discard?"=TRUE ("放弃？")) -> ()  [unwired: 1 in, 1 out]
          }
        }
      }
      frame Error {
        n586 = call <vilib>:"Simple Error Handler.vi"("error in (no error)"=w874) -> ("error out"=w873:errorcluster)  [unwired: 4 in, 4 out]
        n587 = call <vilib>:"Clear Errors.vi"("error in (no error)"=w873) -> ("error out"=w872:errorcluster)  [unwired: 5 in, 1 out]
      }
    }
  }
  n588 = property class="App"() -> ("App.Kind"=w58:T19)  [unwired: 2 in, 2 out]
  n589 = Unregister For Events(event registration refnum=w75, error in=w77) -> (error out=w78:errorcluster)
  n590 = call <vilib>:"Destructor.vi"("error in"=w78, "NotifyIcon"=w74) -> ("error out"=w73:errorcluster)  [unwired: 9 in]
  n591 = call <vilib>:"Simple Error Handler.vi"("error in (no error)"=w73) -> ("error out"=→"错误输出":errorcluster)  [unwired: 4 in, 4 out]
  n592 = case shown="\"Run Time System\"" w58 {
    tunnel: w73 -> [_ _ _ _ _ _ _]
    frame "invalid app kind", Default {
    }
    frame "Development System" {
      n593 = Stop(stop? (T)=TRUE ("可见")) -> ()
    }
    frame "Run Time System" {
      n594 = Quit LabVIEW(quit? (T)=TRUE ("退出？(T)")) -> ()
    }
    frame "Student Edition" {
    }
    frame "Embedded LabVIEW" {
    }
    frame "Evaluation" {
    }
    frame "Custom" {
    }
  }
